vi "Untitled 1 - 22.vi"() -> ()   [LabVIEW 2016]
uses:
  Control 1.ctl
panel:
  out "I F0-ethernet 3":string
  in  "F0-ethernet 3":bool
  out "F0-e 1":bool
  out "I: PZS 2 DOP":string
  out "I: PZS 1 DOP":string
  in  "PZS 2 DOP":bool
  in  "PZS 1 DOP":bool
  out "PZS 2 DOP":bool
  out "PZS 1 DOP":bool
  out "I: BZ1K2W":string
  out "BZ1K2W":bool
  in  "BZ1K2W":bool
  out "I: DZ1K2W":string
  out "DZ1K2W":bool
  in  "DZ1K2W":bool
  out "I: F0-ethernet 4":string
  in  "F0-ethernet 4":bool
  out "F0-e 4":bool
  out "I: BZ2K2W":string
  out "I: DZ2K2W":string
  out "DZ2K2W":bool
  out "BZ2K2W":bool
  in  "BZ2K2W":bool
  in  "DZ2K2W":bool
  out "I: DZ2K1W":string
  out "DZ2K1W":bool
  in  "DZ2K1W":bool
  out "I: BZ2K1W":string
  out "BZ2K1W":bool
  in  "BZ2K1W":bool
  out "I: BZ1K1W":string
  out "BZ1K1W":bool
  in  "BZ1K1W":bool
  out "I: DZ1K1W":string
  out "DZ1K1W":bool
  in  "DZ1K1W":bool
  out "I: F0-ethernet 5":string
  in  "F0-ethernet 5":bool
  out "F0-e 5":bool
  in  "stop":T1
  out "I: BK3":string
  in  "BK3":bool
  out "BK3":bool
  in  "Delay H (0 s)":ext=100.0
  in  "BK3":bool
  in  "Delay G (0 s)":ext=100.0
  in  "BK2":bool
  out "I: BK2":string
  in  "BK 2":bool
  out "BK2":bool
  in  "Delay F (0 s)":ext=100.0
  in  "BK1":bool
  in  "BK1":bool
  out "I: BK1":string
  out "BK1":bool
  out "I F0-ethernet 2":string
  in  "Delay E (0 s)":ext=100.0
  in  "Kamera Y":bool
  out "I: Kamera Y":string
  in  "Kamera Y":bool
  out "Kamera Y":bool
  in  "F0-ethernet 2":bool
  out "F0-e 2":bool
  out "I F0-ethernet 1":string
  in  "F0-ethernet 1":bool
  out "F0-e 3":bool
  out "I: GF":string
  in  "GF":bool
  out "GF":bool
  in  "Delay D (0 s)":ext=100.0
  in  "GF":bool
  out "I: FI":string
  in  "FI":bool
  out "FI":bool
  in  "Delay C (0 s)":ext=100.0
  in  "FI":bool
  in  "F-R VISAR1":bool
  in  "Delay A (0 s)":ext=100.0
  in  "F-R VISAR 4":bool
  out "F-R VISAR 1":bool
  out "I: F-R VISAR 1":string
  in  "F-R VISAR 3":bool
  out "F-R VISAR 2":bool
  out "I: F-R VISAR 2":string
  in  "F-R VISAR2":bool
  in  "Delay B (0 s)":ext=100.0
  out "error out 2":errorcluster
  out "I 0_3":string
  in  "rele 0_6":bool
  out "read buffer 03":string
  out "0_3":bool
  out "read buffer 02":string
  out "read buffer 01":string
  out "error out":errorcluster
  out "VISA resource name out":refnum<visa-resource-name>
  in  "Trigg":bool
  in  "Setup":bool
  in  "Values start":u16(ring)=5 items=["External rising edge"=1, "Single shot internal rising edge"=3, "Single shot"=5]
  # "Current(A)"
  # "FO-ETHERNET ¹1"
  # "VISAR ¹2"
  # "VISAR ¹1"
  # "W ¹2"
  # "Current(A)"
  # "Current(A)"
  # "Current(A)"
  # "FO-ETHERNET ¹4"
  # "1 CHANAL DZ"
  # "2 CHANAL DZ"
  # "Delay (100~1099ns)"
  # "Delay (100~1099ns)"
  # "Current(A)"
  # "Current(A)"
  # "Current(A)"
  # "FO-ETHERNET ¹2"
  # "FORM IMPULSE"
  # "1 CHANAL BZ"
  # "DEEP FRONT"
  # "KAMERA Y"
  # "KAMERA B ¹1"
  # "2 CHANAL BZ"
  # "Current(A)"
  # "Current(A)"
  # "Current(A)"
  # "Current(A)"
  # "Current(A)"
  # "Current(A)"
  # "Delay (100~1099ns)"
  # "Delay (100~1099ns)"
  # "Delay (100~1099ns)"
  # "Delay (100~1099ns)"
  # "W ¹1"
  # "Current(A)"
  # "FO-ETHERNET ¹5"
  # "KAMERA B ¹2"
  # "KAMERA B ¹3"
  # "2 CHANAL DZ"
  # "1 CHANAL DZ"
  # "Current(A)"
  # "Current(A)"
  # "Current(A)"
  # "Current(A)"
  # "Current(A)"
  # "FO-ETHERNET ¹3"
  # "2 CHANAL BZ"
  # "1 CHANAL BZ"
  # "Current(A)"
  # "Current(A)"
  # "PZS ¹1"
  # "PZS ¹2"
  # "Current(A)"
  # "Current(A)"
  # "Delay (100~1099ns)"
  # "Delay (100~1099ns)"
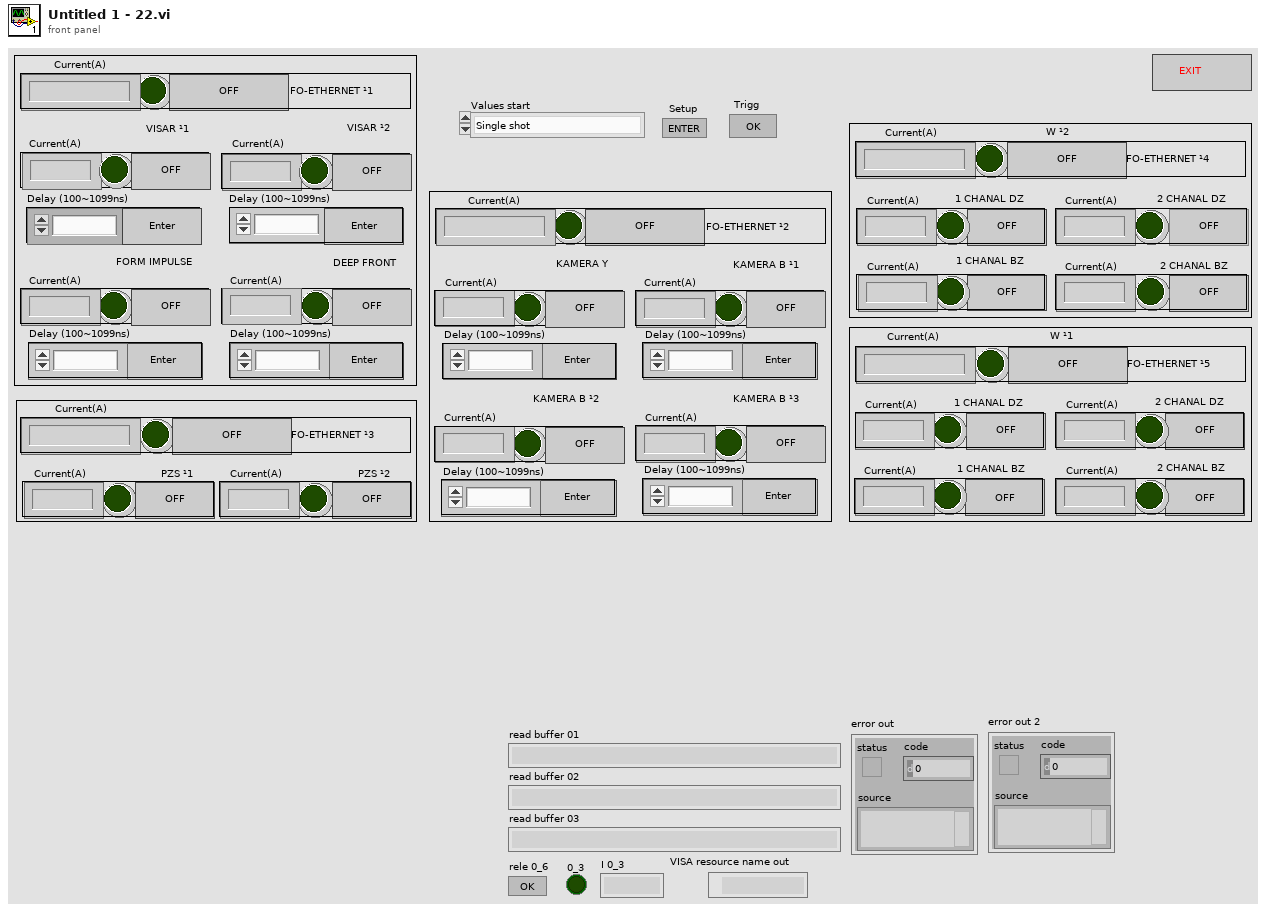
[diagram p1: front panel]
types:
  T1 = typedef "Control 1.ctl" = bool
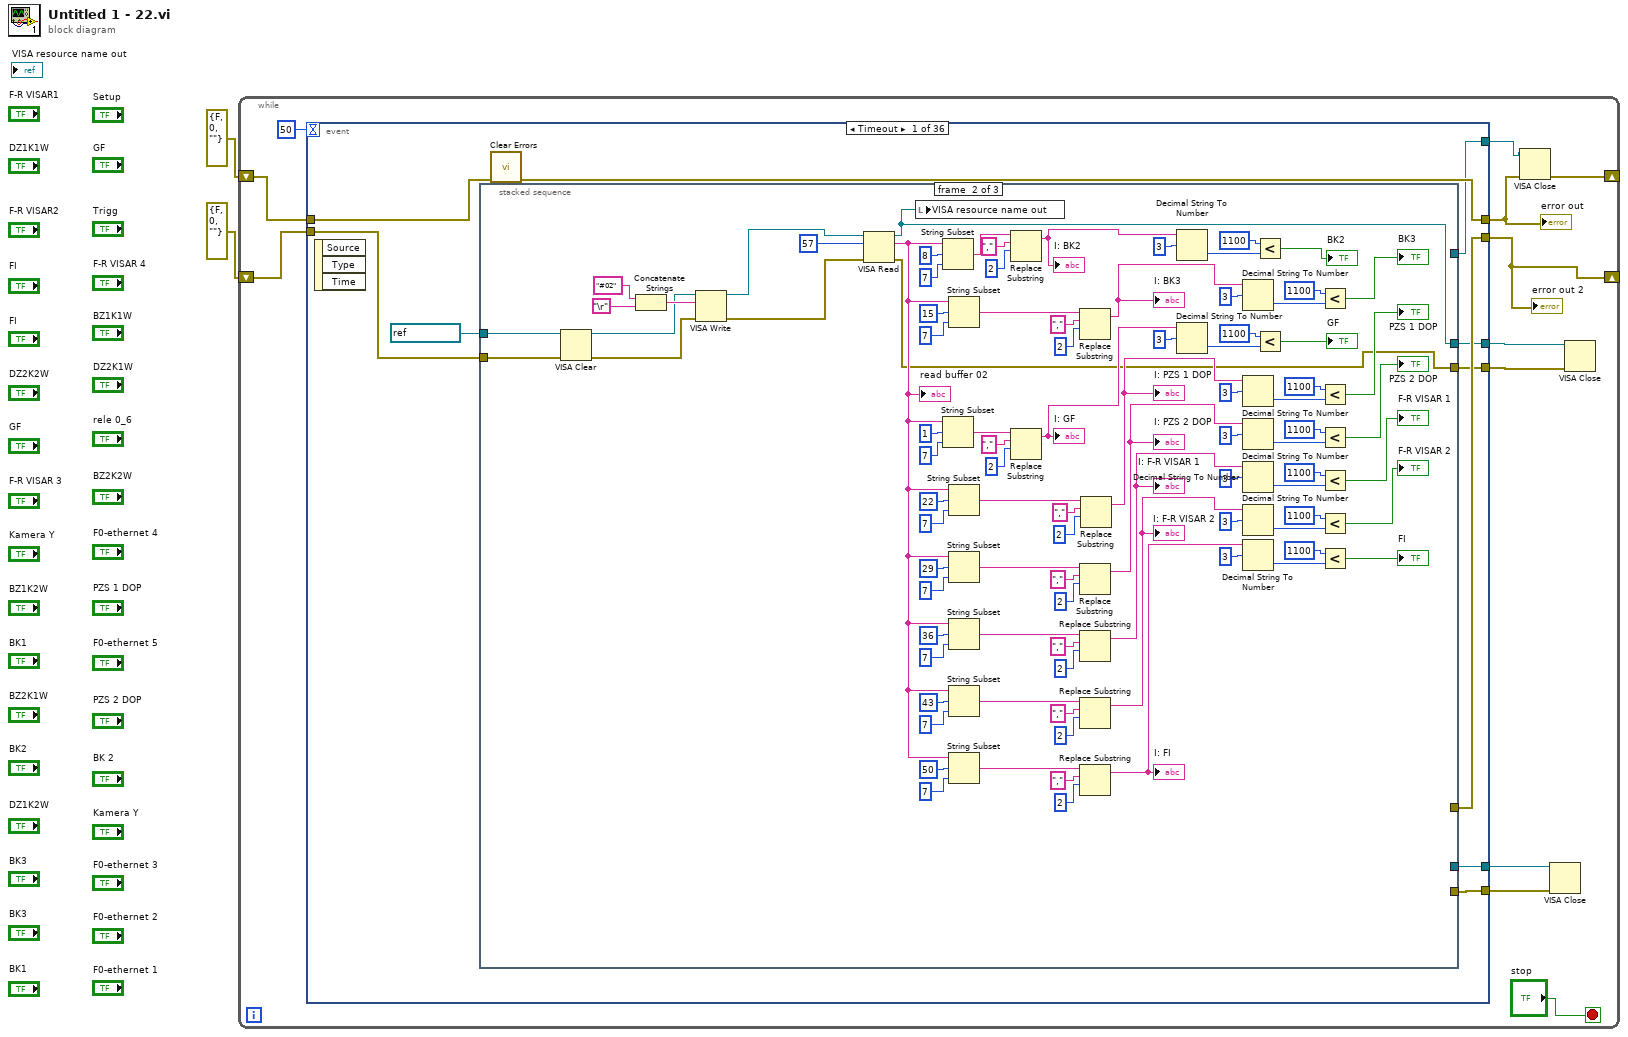
[diagram p0: block diagram]
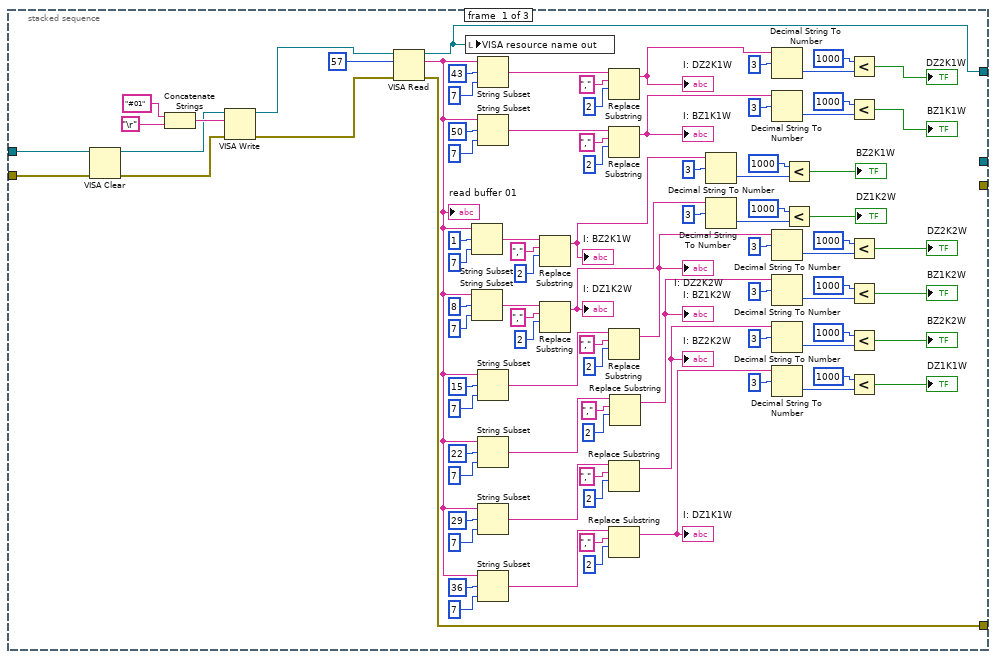
[diagram p2: hidden frame]
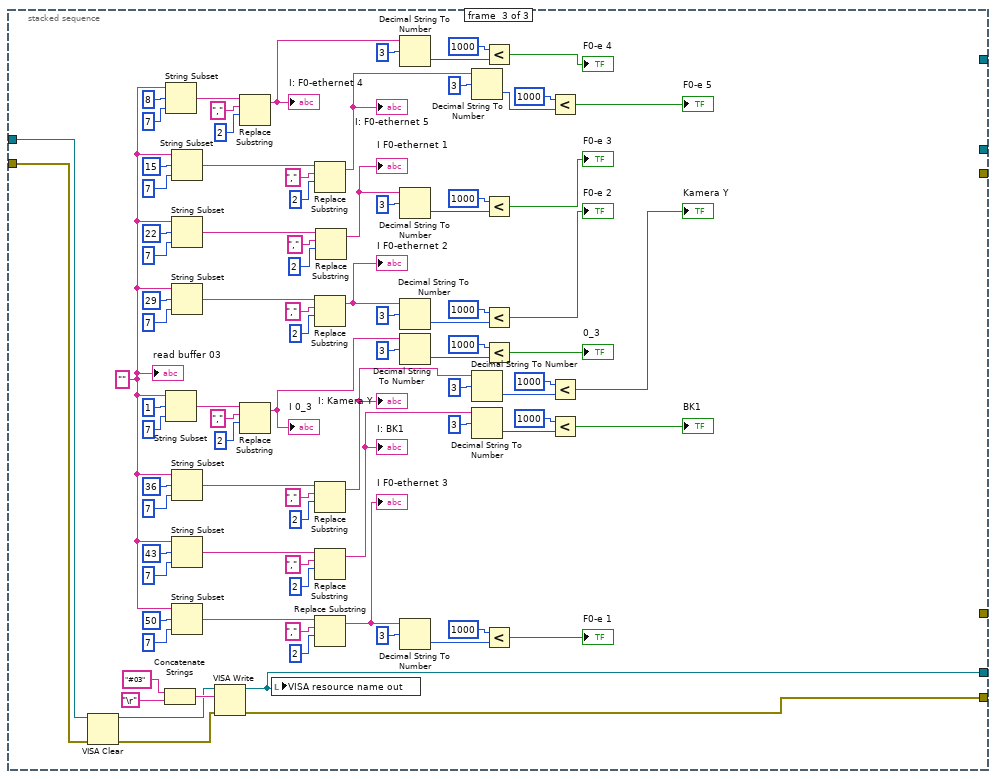
[diagram p3: hidden frame]
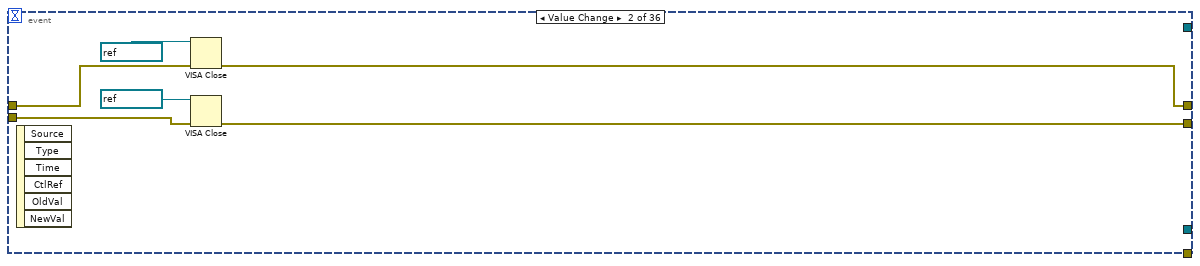
[diagram p4: hidden frame]
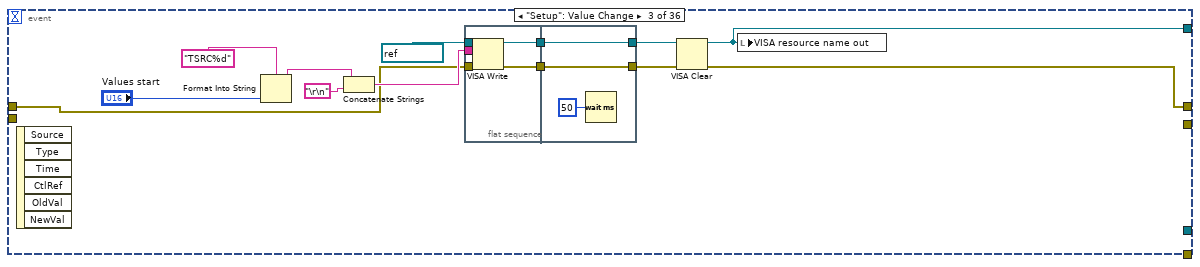
[diagram p5: hidden frame]
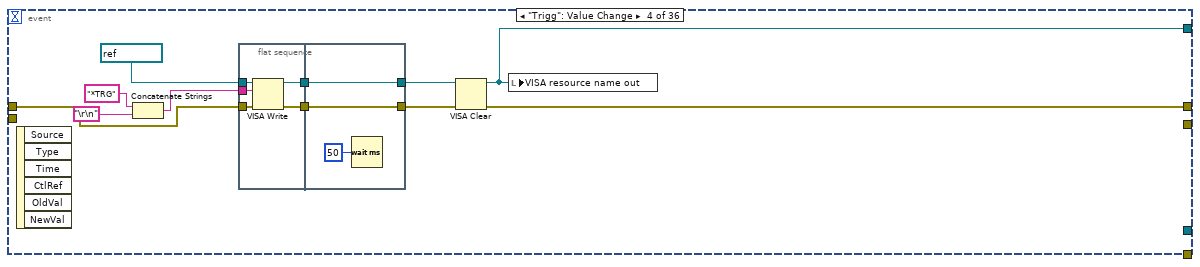
[diagram p6: hidden frame]
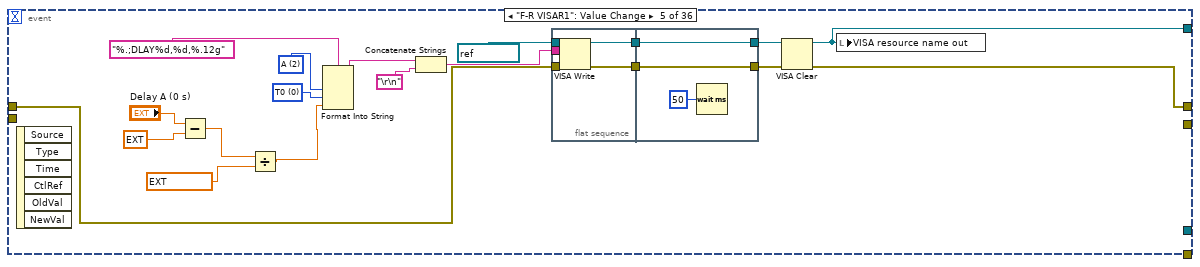
[diagram p7: hidden frame]
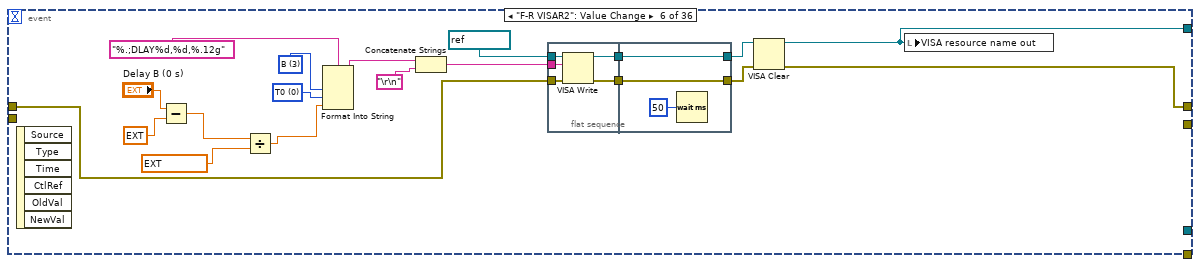
[diagram p8: hidden frame]
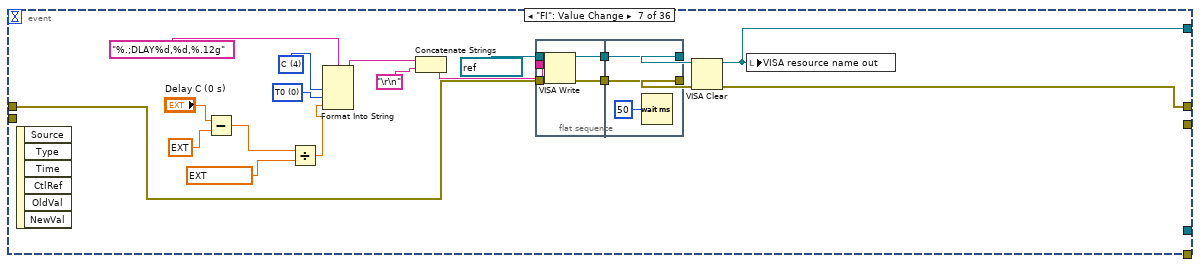
[diagram p9: hidden frame]
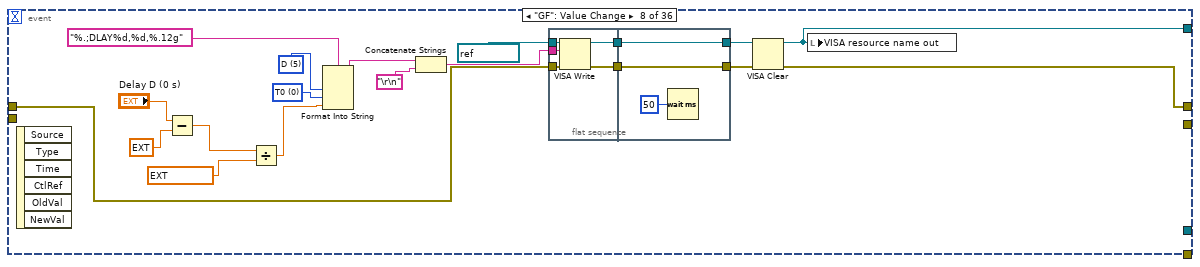
[diagram p10: hidden frame]
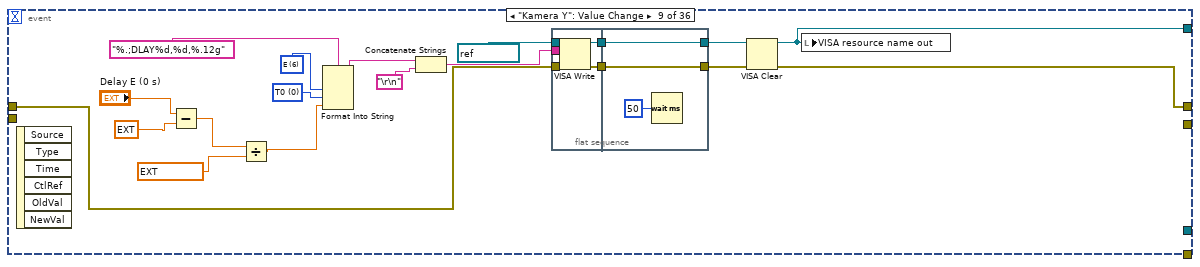
[diagram p11: hidden frame]
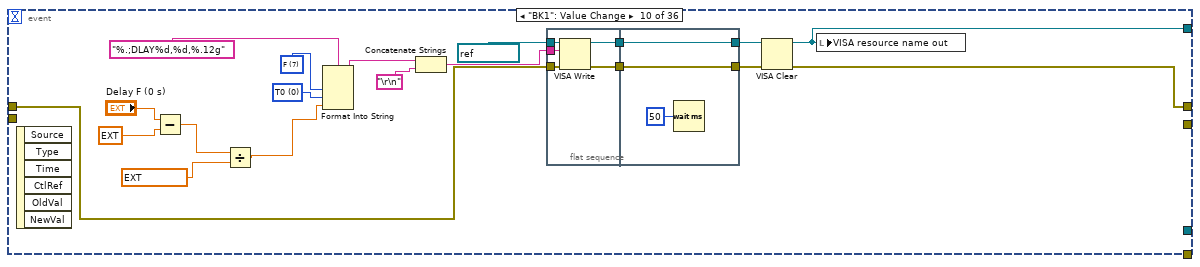
[diagram p12: hidden frame]
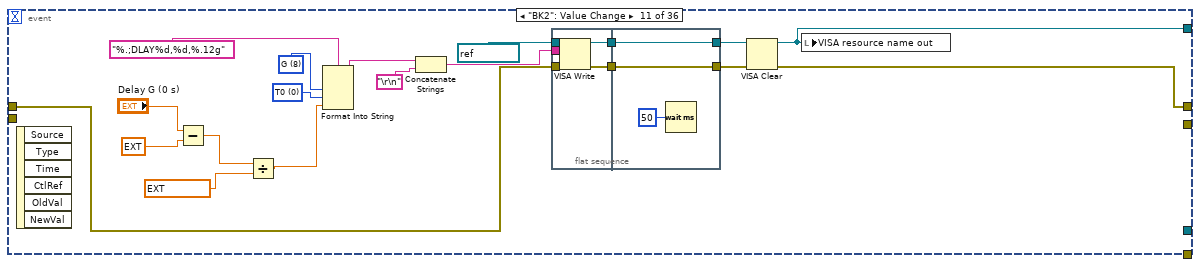
[diagram p13: hidden frame]
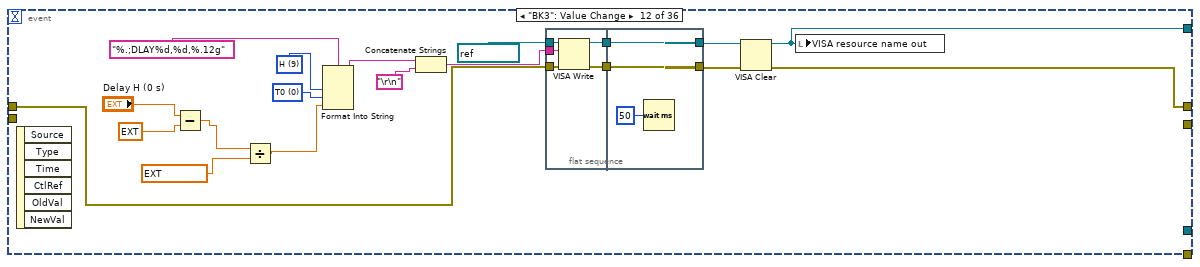
[diagram p14: hidden frame]
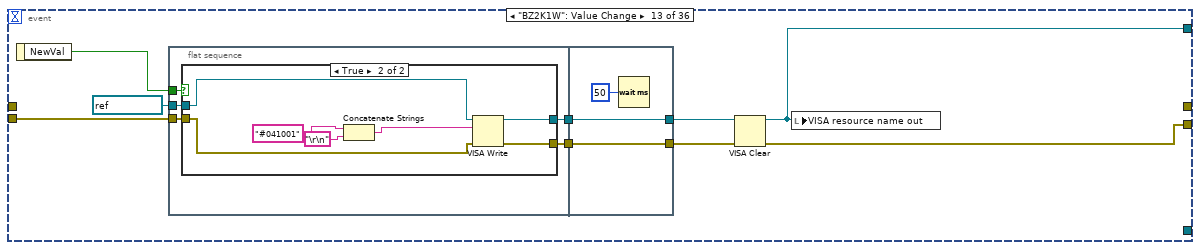
[diagram p15: hidden frame]
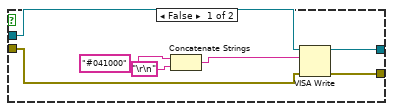
[diagram p16: hidden frame]
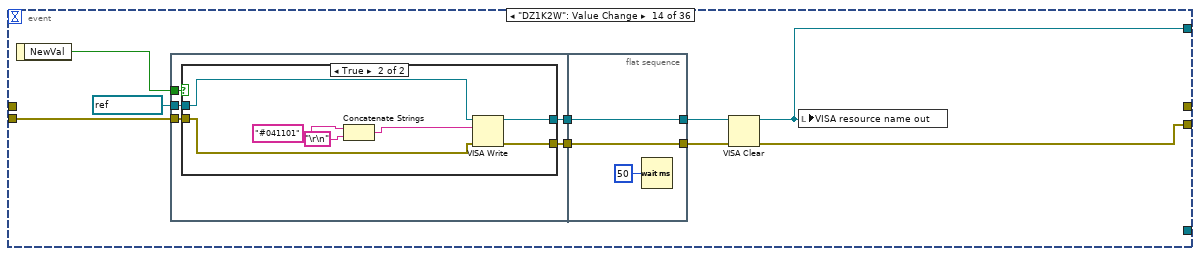
[diagram p17: hidden frame]
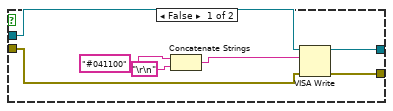
[diagram p18: hidden frame]
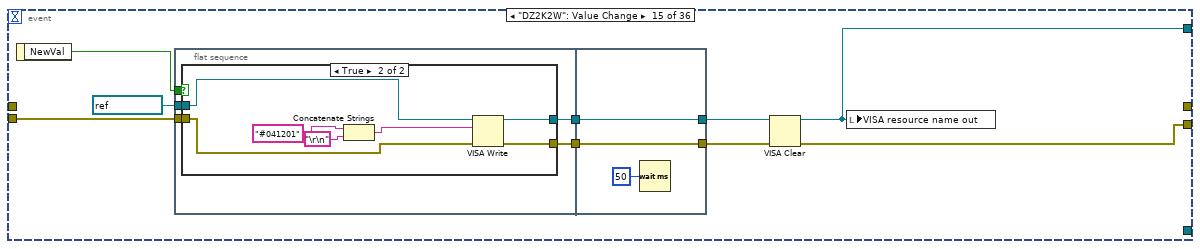
[diagram p19: hidden frame]
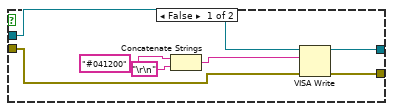
[diagram p20: hidden frame]
diagram:
  n1 = while {
    shift-right: [w11] -> _
    shift-left: errorcluster {"status"=FALSE, "code"=0, "source"=""} ("error out") -> [w14]
    shift-right: [w4] -> _
    shift-left: errorcluster {"status"=FALSE, "code"=0, "source"=""} ("error out") -> [w13]
    stop <- "stop" stop-if-true
    n2 = event shown="[0] Timeout" {
      selector: _ -> [_ _ _ _ _ _ _ _ _ _ _ _ _ _ _ _ _ _ _ _ _ _ _ _ _ _ _ _ _ _ _ _ _ _ _ _]
      dyn-events: _ -> [_ _ _ _ _ _ _ _ _ _ _ _ _ _ _ _ _ _ _ _ _ _ _ _ _ _ _ _ _ _ _ _ _ _ _ _]
      timeout: 50 -> [_ _ _ _ _ _ _ _ _ _ _ _ _ _ _ _ _ _ _ _ _ _ _ _ _ _ _ _ _ _ _ _ _ _ _ _]
      tunnel: [w23 w305 w310 w331 w356 w383 w411 w437 w464 w490 w518 w545 _ _ _ _ _ _ _ _ _ _ _ _ _ _ _ _ _ _ _ _ _ _ _ _] -> w5
      tunnel: w14 -> [w24 w306 w314 w336 w359 w386 w413 w440 w467 w494 w521 w548 _ _ _ _ _ _ _ _ _ _ _ _ _ _ _ _ _ _ _ _ _ _ _ _]
      tunnel: w13 -> [w21 w302 _ _ _ _ _ _ _ _ _ _ w570 w598 w631 w662 w693 w724 w755 w786 w817 w849 w879 w910 w941 w972 w1003 w1035 w1065 w1096 w1127 w1158 w1189 w1220 w1251 w1282]
      tunnel: [w20 w301 _ _ _ _ _ _ _ _ _ _ w566 w597 w628 w659 w691 w721 w753 w783 w814 w845 w876 w907 w938 w969 w1000 w1031 w1062 w1093 w1124 w1155 w1186 w1217 w1248 w1279] -> w4
      tunnel: [w19 _ w307 w328 w352 w379 w406 w433 w460 w487 w514 w541 w563 w594 w625 w656 w687 w718 w749 w780 w811 w842 w873 w904 w935 w966 w997 w1028 w1059 w1090 w1121 w1152 w1183 w1214 w1245 w1276] -> w10
      tunnel: [w18 _ _ _ _ _ _ _ _ _ _ _ _ _ _ _ _ _ _ _ _ _ _ _ _ _ _ _ _ _ _ _ _ _ _ _] -> w9
      tunnel: [w17 _ _ _ _ _ _ _ _ _ _ _ _ _ _ _ _ _ _ _ _ _ _ _ _ _ _ _ _ _ _ _ _ _ _ _] -> w8
      tunnel: [w16 _ _ _ _ _ _ _ _ _ _ _ _ _ _ _ _ _ _ _ _ _ _ _ _ _ _ _ _ _ _ _ _ _ _ _] -> w7
      tunnel: [w15 _ _ _ _ _ _ _ _ _ _ _ _ _ _ _ _ _ _ _ _ _ _ _ _ _ _ _ _ _ _ _ _ _ _ _] -> w6
      event Timeout {
        n3 = event-data() -> ()  [unwired: 1 in, 3 out]
        n4 = stacked-sequence {
          tunnel: refnum<visa-resource-name> "COM1" ("VISA resource name") -> [w29 w121 w234]
          tunnel: [w71 _ _] -> w20
          tunnel: w21 -> [w28 w123 w230]
          tunnel: [w25 _ _] -> w19
          tunnel: [_ w119 _] -> w18
          tunnel: [_ w118 _] -> w17
          tunnel: [_ _ w212] -> w16
          tunnel: [_ _ w211] -> w15
          frame #0 {
            n5 = VISA Clear(VISA resource name=w29, error in (no error)=w28) -> (VISA resource name out=w26:refnum<visa-resource-name>, error out=w27:errorcluster)
            n6 = Concatenate Strings("#01" ("string"), "\r") -> (w117:string)
            n7 = VISA Write(VISA resource name=w26, write buffer=w117, error in (no error)=w27) -> (VISA resource name out=w74:refnum<visa-resource-name>, error out=w73:errorcluster)  [unwired: 1 out]
            n8 = VISA Read(VISA resource name=w74, byte count=u32 57, error in (no error)=w73) -> (VISA resource name out=w25:refnum<visa-resource-name>, read buffer=w46:string, error out=w71:errorcluster)  [unwired: 1 out]
            "read buffer 01" <- w46
            n9 = local write "VISA resource name out"(w25) -> ()
            n10 = String Subset(string=w46, offset (0)=1, length (rest)=7 ("length (rest)")) -> (substring=w91:string)
            n11 = String Subset(string=w46, offset (0)=8, length (rest)=7 ("length (rest)")) -> (substring=w96:string)
            n12 = String Subset(string=w46, offset (0)=43, length (rest)=7 ("length (rest)")) -> (substring=w111:string)
            n13 = String Subset(string=w46, offset (0)=50, length (rest)=7 ("length (rest)")) -> (substring=w114:string)
            n14 = String Subset(string=w46, offset (0)=15, length (rest)=7 ("length (rest)")) -> (substring=w99:string)
            n15 = String Subset(string=w46, offset (0)=22, length (rest)=7 ("length (rest)")) -> (substring=w102:string)
            n16 = String Subset(string=w46, offset (0)=29, length (rest)=7 ("length (rest)")) -> (substring=w105:string)
            n17 = String Subset(string=w46, offset (0)=36, length (rest)=7 ("length (rest)")) -> (substring=w108:string)
            n18 = Replace Substring(3:2 ("offset (0)"), 4:"," ("substring (\"\")"), 5:w91) -> (1:w45:string)  [unwired: 1 in, 1 out]
            "I: BZ2K1W" <- w45
            n19 = Replace Substring(3:2 ("offset (0)"), 4:"," ("substring (\"\")"), 5:w96) -> (1:w43:string)  [unwired: 1 in, 1 out]
            "I: DZ1K2W" <- w43
            n20 = Replace Substring(3:2 ("offset (0)"), 4:"," ("substring (\"\")"), 5:w111) -> (1:w32:string)  [unwired: 1 in, 1 out]
            "I: DZ2K1W" <- w32
            n21 = Replace Substring(3:2 ("offset (0)"), 4:"," ("substring (\"\")"), 5:w114) -> (1:w31:string)  [unwired: 1 in, 1 out]
            "I: BZ1K1W" <- w31
            n22 = Replace Substring(3:2 ("offset (0)"), 4:"," ("substring (\"\")"), 5:w99) -> (1:w41:string)  [unwired: 1 in, 1 out]
            "I: DZ2K2W" <- w41
            n23 = Replace Substring(3:2 ("offset (0)"), 4:"," ("substring (\"\")"), 5:w105) -> (1:w37:string)  [unwired: 1 in, 1 out]
            "I: BZ2K2W" <- w37
            n24 = Replace Substring(3:2 ("offset (0)"), 4:"," ("substring (\"\")"), 5:w108) -> (1:w34:string)  [unwired: 1 in, 1 out]
            "I: DZ1K1W" <- w34
            n25 = Replace Substring(3:2 ("offset (0)"), 4:"," ("substring (\"\")"), 5:w102) -> (1:w39:string)  [unwired: 1 in, 1 out]
            "I: BZ1K2W" <- w39
            n26 = Decimal String To Number(string=w45, offset=3) -> (number=w54:i32)  [unwired: 1 in, 1 out]
            n27 = Decimal String To Number(string=w43, offset=3) -> (number=w57:i32)  [unwired: 1 in, 1 out]
            n28 = Decimal String To Number(string=w32, offset=3) -> (number=w51:i32)  [unwired: 1 in, 1 out]
            n29 = Decimal String To Number(string=w31, offset=3) -> (number=w48:i32)  [unwired: 1 in, 1 out]
            n30 = Decimal String To Number(string=w41, offset=3) -> (number=w60:i32)  [unwired: 1 in, 1 out]
            n31 = Decimal String To Number(string=w39, offset=3) -> (number=w63:i32)  [unwired: 1 in, 1 out]
            n32 = Decimal String To Number(string=w37, offset=3) -> (number=w66:i32)  [unwired: 1 in, 1 out]
            n33 = Decimal String To Number(string=w34, offset=3) -> (number=w69:i32)  [unwired: 1 in, 1 out]
            n34 = Less?(x=1000, y=w54) -> (x < y?=→"BZ2K1W":bool)
            n35 = Less?(x=1000, y=w57) -> (x < y?=→"DZ1K2W":bool)
            n36 = Less?(x=1000, y=w51) -> (x < y?=→"DZ2K1W":bool)
            n37 = Less?(x=1000, y=w48) -> (x < y?=→"BZ1K1W":bool)
            n38 = Less?(x=1000, y=w60) -> (x < y?=→"DZ2K2W":bool)
            n39 = Less?(x=1000, y=w63) -> (x < y?=→"BZ1K2W":bool)
            n40 = Less?(x=1000, y=w66) -> (x < y?=→"BZ2K2W":bool)
            n41 = Less?(x=1000, y=w69) -> (x < y?=→"DZ1K1W":bool)
          }
          frame #1 {
            n42 = VISA Clear(VISA resource name=w121, error in (no error)=w123) -> (VISA resource name out=w120:refnum<visa-resource-name>, error out=w122:errorcluster)
            n43 = Concatenate Strings("#02" ("string"), "\r") -> (w210:string)
            n44 = VISA Write(VISA resource name=w120, write buffer=w210, error in (no error)=w122) -> (VISA resource name out=w167:refnum<visa-resource-name>, error out=w166:errorcluster)  [unwired: 1 out]
            n45 = VISA Read(VISA resource name=w167, byte count=u32 57, error in (no error)=w166) -> (VISA resource name out=w119:refnum<visa-resource-name>, read buffer=w140:string, error out=w118:errorcluster)  [unwired: 1 out]
            "read buffer 02" <- w140
            n46 = local write "VISA resource name out"(w119) -> ()
            n47 = String Subset(string=w140, offset (0)=8, length (rest)=7 ("length (rest)")) -> (substring=w189:string)
            n48 = String Subset(string=w140, offset (0)=1, length (rest)=7 ("length (rest)")) -> (substring=w184:string)
            n49 = String Subset(string=w140, offset (0)=15, length (rest)=7 ("length (rest)")) -> (substring=w192:string)
            n50 = String Subset(string=w140, offset (0)=22, length (rest)=7 ("length (rest)")) -> (substring=w195:string)
            n51 = String Subset(string=w140, offset (0)=29, length (rest)=7 ("length (rest)")) -> (substring=w198:string)
            n52 = String Subset(string=w140, offset (0)=36, length (rest)=7 ("length (rest)")) -> (substring=w201:string)
            n53 = String Subset(string=w140, offset (0)=43, length (rest)=7 ("length (rest)")) -> (substring=w204:string)
            n54 = String Subset(string=w140, offset (0)=50, length (rest)=7 ("length (rest)")) -> (substring=w207:string)
            n55 = Replace Substring(3:2 ("offset (0)"), 4:"," ("substring (\"\")"), 5:w189) -> (1:w136:string)  [unwired: 1 in, 1 out]
            "I: BK2" <- w136
            n56 = Replace Substring(3:2 ("offset (0)"), 4:"," ("substring (\"\")"), 5:w184) -> (1:w138:string)  [unwired: 1 in, 1 out]
            "I: GF" <- w138
            n57 = Replace Substring(3:2 ("offset (0)"), 4:"," ("substring (\"\")"), 5:w192) -> (1:w135:string)  [unwired: 1 in, 1 out]
            "I: BK3" <- w135
            n58 = Replace Substring(3:2 ("offset (0)"), 4:"," ("substring (\"\")"), 5:w198) -> (1:w130:string)  [unwired: 1 in, 1 out]
            "I: PZS 2 DOP" <- w130
            n59 = Replace Substring(3:2 ("offset (0)"), 4:"," ("substring (\"\")"), 5:w201) -> (1:w128:string)  [unwired: 1 in, 1 out]
            "I: F-R VISAR 1" <- w128
            n60 = Replace Substring(3:2 ("offset (0)"), 4:"," ("substring (\"\")"), 5:w204) -> (1:w127:string)  [unwired: 1 in, 1 out]
            "I: F-R VISAR 2" <- w127
            n61 = Replace Substring(3:2 ("offset (0)"), 4:"," ("substring (\"\")"), 5:w207) -> (1:w126:string)  [unwired: 1 in, 1 out]
            "I: FI" <- w126
            n62 = Replace Substring(3:2 ("offset (0)"), 4:"," ("substring (\"\")"), 5:w195) -> (1:w133:string)  [unwired: 1 in, 1 out]
            "I: PZS 1 DOP" <- w133
            n63 = Decimal String To Number(string=w136, offset=3) -> (number=w151:i32)  [unwired: 1 in, 1 out]
            n64 = Decimal String To Number(string=w138, offset=3) -> (number=w148:i32)  [unwired: 1 in, 1 out]
            n65 = Decimal String To Number(string=w135, offset=3) -> (number=w154:i32)  [unwired: 1 in, 1 out]
            n66 = Decimal String To Number(string=w133, offset=3) -> (number=w157:i32)  [unwired: 1 in, 1 out]
            n67 = Decimal String To Number(string=w130, offset=3) -> (number=w160:i32)  [unwired: 1 in, 1 out]
            n68 = Decimal String To Number(string=w128, offset=3) -> (number=w163:i32)  [unwired: 1 in, 1 out]
            n69 = Decimal String To Number(string=w127, offset=3) -> (number=w145:i32)  [unwired: 1 in, 1 out]
            n70 = Decimal String To Number(string=w126, offset=3) -> (number=w142:i32)  [unwired: 1 in, 1 out]
            n71 = Less?(x=1100, y=w151) -> (x < y?=→"BK2":bool)
            n72 = Less?(x=1100, y=w148) -> (x < y?=→"GF":bool)
            n73 = Less?(x=1100, y=w154) -> (x < y?=→"BK3":bool)
            n74 = Less?(x=1100, y=w157) -> (x < y?=→"PZS 1 DOP":bool)
            n75 = Less?(x=1100, y=w160) -> (x < y?=→"PZS 2 DOP":bool)
            n76 = Less?(x=1100, y=w163) -> (x < y?=→"F-R VISAR 1":bool)
            n77 = Less?(x=1100, y=w145) -> (x < y?=→"F-R VISAR 2":bool)
            n78 = Less?(x=1100, y=w142) -> (x < y?=→"FI":bool)
          }
          frame #2 {
            w229 = "" ("string")
            n79 = VISA Clear(VISA resource name=w234, error in (no error)=w230) -> (VISA resource name out=w232:refnum<visa-resource-name>, error out=w233:errorcluster)
            n80 = Concatenate Strings("#03" ("string"), "\r") -> (w300:string)
            n81 = String Subset(string=w229, offset (0)=8, length (rest)=7 ("length (rest)")) -> (substring=w279:string)
            n82 = String Subset(string=w229, offset (0)=1, length (rest)=7 ("length (rest)")) -> (substring=w231:string)
            n83 = String Subset(string=w229, offset (0)=15, length (rest)=7 ("length (rest)")) -> (substring=w282:string)
            n84 = String Subset(string=w229, offset (0)=22, length (rest)=7 ("length (rest)")) -> (substring=w285:string)
            n85 = String Subset(string=w229, offset (0)=29, length (rest)=7 ("length (rest)")) -> (substring=w288:string)
            n86 = String Subset(string=w229, offset (0)=36, length (rest)=7 ("length (rest)")) -> (substring=w291:string)
            n87 = String Subset(string=w229, offset (0)=43, length (rest)=7 ("length (rest)")) -> (substring=w294:string)
            n88 = String Subset(string=w229, offset (0)=50, length (rest)=7 ("length (rest)")) -> (substring=w297:string)
            n89 = VISA Write(VISA resource name=w232, write buffer=w300, error in (no error)=w233) -> (VISA resource name out=w211:refnum<visa-resource-name>, error out=w212:errorcluster)  [unwired: 1 out]
            n90 = Replace Substring(3:2 ("offset (0)"), 4:"," ("substring (\"\")"), 5:w279) -> (1:w226:string)  [unwired: 1 in, 1 out]
            "I: F0-ethernet 4" <- w226
            n91 = Replace Substring(3:2 ("offset (0)"), 4:"," ("substring (\"\")"), 5:w231) -> (1:w228:string)  [unwired: 1 in, 1 out]
            "I 0_3" <- w228
            n92 = local write "VISA resource name out"(w211) -> ()
            n93 = Replace Substring(3:2 ("offset (0)"), 4:"," ("substring (\"\")"), 5:w282) -> (1:w224:string)  [unwired: 1 in, 1 out]
            "I: F0-ethernet 5" <- w224
            n94 = Replace Substring(3:2 ("offset (0)"), 4:"," ("substring (\"\")"), 5:w288) -> (1:w219:string)  [unwired: 1 in, 1 out]
            "I F0-ethernet 2" <- w219
            n95 = Replace Substring(3:2 ("offset (0)"), 4:"," ("substring (\"\")"), 5:w291) -> (1:w217:string)  [unwired: 1 in, 1 out]
            "I: Kamera Y" <- w217
            n96 = Replace Substring(3:2 ("offset (0)"), 4:"," ("substring (\"\")"), 5:w294) -> (1:w215:string)  [unwired: 1 in, 1 out]
            "I: BK1" <- w215
            n97 = Replace Substring(3:2 ("offset (0)"), 4:"," ("substring (\"\")"), 5:w297) -> (1:w213:string)  [unwired: 1 in, 1 out]
            "I F0-ethernet 3" <- w213
            n98 = Replace Substring(3:2 ("offset (0)"), 4:"," ("substring (\"\")"), 5:w285) -> (1:w222:string)  [unwired: 1 in, 1 out]
            "I F0-ethernet 1" <- w222
            n99 = Decimal String To Number(string=w226, offset=3) -> (number=w245:i32)  [unwired: 1 in, 1 out]
            n100 = Decimal String To Number(string=w222, offset=3) -> (number=w251:i32)  [unwired: 1 in, 1 out]
            n101 = Decimal String To Number(string=w219, offset=3) -> (number=w254:i32)  [unwired: 1 in, 1 out]
            n102 = Decimal String To Number(string=w228, offset=3) -> (number=w242:i32)  [unwired: 1 in, 1 out]
            n103 = Decimal String To Number(string=w213, offset=3) -> (number=w236:i32)  [unwired: 1 in, 1 out]
            n104 = Decimal String To Number(string=w224, offset=3) -> (number=w248:i32)  [unwired: 1 in, 1 out]
            n105 = Decimal String To Number(string=w217, offset=3) -> (number=w257:i32)  [unwired: 1 in, 1 out]
            n106 = Decimal String To Number(string=w215, offset=3) -> (number=w239:i32)  [unwired: 1 in, 1 out]
            n107 = Less?(x=1000, y=w245) -> (x < y?=→"F0-e 4":bool)
            n108 = Less?(x=1000, y=w251) -> (x < y?=→"F0-e 3":bool)
            n109 = Less?(x=1000, y=w254) -> (x < y?=→"F0-e 2":bool)
            n110 = Less?(x=1000, y=w242) -> (x < y?=→"0_3":bool)
            n111 = Less?(x=1000, y=w236) -> (x < y?=→"F0-e 1":bool)
            n112 = Less?(x=1000, y=w248) -> (x < y?=→"F0-e 5":bool)
            n113 = Less?(x=1000, y=w257) -> (x < y?=→"Kamera Y":bool)
            n114 = Less?(x=1000, y=w239) -> (x < y?=→"BK1":bool)
            "read buffer 03" <- w229
          }
        }
        n115 = call <vilib>:"Clear Errors.vi"("error in (no error)"=w24) -> ("error out"=w23:errorcluster)  [unwired: 5 in, 1 out]
      }
      event Value Change {
        n116 = event-data() -> ()  [unwired: 1 in, 6 out]
        n117 = VISA Close(VISA resource name=refnum<visa-resource-name> "DG645", error in (no error)=w306) -> (error out=w305:errorcluster)
        n118 = VISA Close(VISA resource name=refnum<visa-resource-name> "COM1", error in (no error)=w302) -> (error out=w301:errorcluster)
      }
      event "Setup": Value Change {
        n119 = event-data() -> ()  [unwired: 1 in, 6 out]
        n120 = Format Into String(format string="TSRC%d", "Values start") -> (resulting string=w317:string)  [unwired: 2 in, 1 out]
        n121 = Concatenate Strings(w317, "\r\n") -> (w319:string)
        n122 = flat-sequence {
          tunnel: w319 -> [w324]
          tunnel: w314 -> [w323]
          tunnel: refnum<visa-resource-name> "DG645" ("VISA resource name") -> [w322]
          tunnel: [w321] -> w309
          tunnel: [w320] -> w308
          tunnel: [w326] -> w311
          tunnel: [w327] -> w312
          tunnel: w309 -> [w327]
          tunnel: w308 -> [w326]
          frame #0 {
            n123 = VISA Write(VISA resource name=w322, write buffer=w324, error in (no error)=w323) -> (VISA resource name out=w320:refnum<visa-resource-name>, error out=w321:errorcluster)  [unwired: 1 out]
          }
          frame #1 {
            n124 = Wait (ms)(milliseconds to wait=u32 50) -> ()  [unwired: 1 out]
          }
        }
        n125 = VISA Clear(VISA resource name=w311, error in (no error)=w312) -> (VISA resource name out=w307:refnum<visa-resource-name>, error out=w310:errorcluster)
        n126 = local write "VISA resource name out"(w307) -> ()
      }
      event "Trigg": Value Change {
        n127 = event-data() -> ()  [unwired: 1 in, 6 out]
        n128 = Concatenate Strings("*TRG" ("string"), "\r\n") -> (w337:string)
        n129 = flat-sequence {
          tunnel: w337 -> [w343]
          tunnel: w336 -> [w342]
          tunnel: refnum<visa-resource-name> "DG645" ("VISA resource name") -> [w341]
          tunnel: [w340] -> w330
          tunnel: [w339] -> w329
          tunnel: [w345] -> w332
          tunnel: [w346] -> w333
          tunnel: w330 -> [w346]
          tunnel: w329 -> [w345]
          frame #0 {
            n130 = VISA Write(VISA resource name=w341, write buffer=w343, error in (no error)=w342) -> (VISA resource name out=w339:refnum<visa-resource-name>, error out=w340:errorcluster)  [unwired: 1 out]
          }
          frame #1 {
            n131 = Wait (ms)(milliseconds to wait=u32 50) -> ()  [unwired: 1 out]
          }
        }
        n132 = VISA Clear(VISA resource name=w332, error in (no error)=w333) -> (VISA resource name out=w328:refnum<visa-resource-name>, error out=w331:errorcluster)
        n133 = local write "VISA resource name out"(w328) -> ()
      }
      event "F-R VISAR1": Value Change {
        w360 = u16 0 items=["T0"=0, "A"=2, "B"=3, "C"=4, "D"=5, "E"=6, "F"=7, "G"=8, "H"=9] ("Reference Channel (0:T0)")
        w364 = u16 2 items=["A"=2, "B"=3, "C"=4, "D"=5, "E"=6, "F"=7, "G"=8, "H"=9] ("Channel to Modify (2:A)")
        n134 = event-data() -> ()  [unwired: 1 in, 6 out]
        n135 = Subtract(x="Delay A (0 s)", y=ext 100.0) -> (x-y=w347:ext)
        n136 = Divide(x=w347, y=ext 1000000000.0) -> (x/y=w350:ext)
        n137 = Format Into String(format string="%.;DLAY%d,%d,%.12g" ("Set Delay Command"), w364, w360, w350) -> (resulting string=w363:string)  [unwired: 2 in, 1 out]
        n138 = Concatenate Strings(w363, "\r\n") -> (w362:string)
        n139 = flat-sequence {
          tunnel: w362 -> [w370]
          tunnel: w359 -> [w369]
          tunnel: refnum<visa-resource-name> "DG645" ("VISA resource name") -> [w368]
          tunnel: [w367] -> w354
          tunnel: [w366] -> w353
          tunnel: [w372] -> w355
          tunnel: [w373] -> w357
          tunnel: w354 -> [w373]
          tunnel: w353 -> [w372]
          frame #0 {
            n140 = VISA Write(VISA resource name=w368, write buffer=w370, error in (no error)=w369) -> (VISA resource name out=w366:refnum<visa-resource-name>, error out=w367:errorcluster)  [unwired: 1 out]
          }
          frame #1 {
            n141 = Wait (ms)(milliseconds to wait=u32 50) -> ()  [unwired: 1 out]
          }
        }
        n142 = VISA Clear(VISA resource name=w355, error in (no error)=w357) -> (VISA resource name out=w352:refnum<visa-resource-name>, error out=w356:errorcluster)
        n143 = local write "VISA resource name out"(w352) -> ()
      }
      event "F-R VISAR2": Value Change {
        w387 = u16 0 items=["T0"=0, "A"=2, "B"=3, "C"=4, "D"=5, "E"=6, "F"=7, "G"=8, "H"=9] ("Reference Channel (0:T0)")
        w391 = u16 3 items=["A"=2, "B"=3, "C"=4, "D"=5, "E"=6, "F"=7, "G"=8, "H"=9] ("Channel to Modify (2:A)")
        n144 = event-data() -> ()  [unwired: 1 in, 6 out]
        n145 = Subtract(x="Delay B (0 s)", y=ext 100.0) -> (x-y=w374:ext)
        n146 = Divide(x=w374, y=ext 1000000000.0) -> (x/y=w377:ext)
        n147 = Format Into String(format string="%.;DLAY%d,%d,%.12g" ("Set Delay Command"), w391, w387, w377) -> (resulting string=w390:string)  [unwired: 2 in, 1 out]
        n148 = Concatenate Strings(w390, "\r\n") -> (w389:string)
        n149 = flat-sequence {
          tunnel: w389 -> [w397]
          tunnel: w386 -> [w396]
          tunnel: refnum<visa-resource-name> "DG645" ("VISA resource name") -> [w395]
          tunnel: [w394] -> w381
          tunnel: [w393] -> w380
          tunnel: [w399] -> w382
          tunnel: [w400] -> w384
          tunnel: w381 -> [w400]
          tunnel: w380 -> [w399]
          frame #0 {
            n150 = VISA Write(VISA resource name=w395, write buffer=w397, error in (no error)=w396) -> (VISA resource name out=w393:refnum<visa-resource-name>, error out=w394:errorcluster)  [unwired: 1 out]
          }
          frame #1 {
            n151 = Wait (ms)(milliseconds to wait=u32 50) -> ()  [unwired: 1 out]
          }
        }
        n152 = VISA Clear(VISA resource name=w382, error in (no error)=w384) -> (VISA resource name out=w379:refnum<visa-resource-name>, error out=w383:errorcluster)
        n153 = local write "VISA resource name out"(w379) -> ()
      }
      event "FI": Value Change {
        w414 = u16 0 items=["T0"=0, "A"=2, "B"=3, "C"=4, "D"=5, "E"=6, "F"=7, "G"=8, "H"=9] ("Reference Channel (0:T0)")
        w418 = u16 4 items=["A"=2, "B"=3, "C"=4, "D"=5, "E"=6, "F"=7, "G"=8, "H"=9] ("Channel to Modify (2:A)")
        n154 = event-data() -> ()  [unwired: 1 in, 6 out]
        n155 = Subtract(x="Delay C (0 s)", y=ext 100.0) -> (x-y=w402:ext)
        n156 = Divide(x=w402, y=ext 1000000000.0) -> (x/y=w403:ext)
        n157 = Format Into String(format string="%.;DLAY%d,%d,%.12g" ("Set Delay Command"), w418, w414, w403) -> (resulting string=w417:string)  [unwired: 2 in, 1 out]
        n158 = Concatenate Strings(w417, "\r\n") -> (w416:string)
        n159 = flat-sequence {
          tunnel: w416 -> [w424]
          tunnel: w413 -> [w423]
          tunnel: refnum<visa-resource-name> "DG645" ("VISA resource name") -> [w422]
          tunnel: [w421] -> w408
          tunnel: [w420] -> w407
          tunnel: [w426] -> w409
          tunnel: [w427] -> w410
          tunnel: w408 -> [w427]
          tunnel: w407 -> [w426]
          frame #0 {
            n160 = VISA Write(VISA resource name=w422, write buffer=w424, error in (no error)=w423) -> (VISA resource name out=w420:refnum<visa-resource-name>, error out=w421:errorcluster)  [unwired: 1 out]
          }
          frame #1 {
            n161 = Wait (ms)(milliseconds to wait=u32 50) -> ()  [unwired: 1 out]
          }
        }
        n162 = VISA Clear(VISA resource name=w409, error in (no error)=w410) -> (VISA resource name out=w406:refnum<visa-resource-name>, error out=w411:errorcluster)
        n163 = local write "VISA resource name out"(w406) -> ()
      }
      event "GF": Value Change {
        w441 = u16 0 items=["T0"=0, "A"=2, "B"=3, "C"=4, "D"=5, "E"=6, "F"=7, "G"=8, "H"=9] ("Reference Channel (0:T0)")
        w445 = u16 5 items=["A"=2, "B"=3, "C"=4, "D"=5, "E"=6, "F"=7, "G"=8, "H"=9] ("Channel to Modify (2:A)")
        n164 = event-data() -> ()  [unwired: 1 in, 6 out]
        n165 = Subtract(x="Delay D (0 s)", y=ext 100.0) -> (x-y=w430:ext)
        n166 = Divide(x=w430, y=ext 1000000000.0) -> (x/y=w428:ext)
        n167 = Format Into String(format string="%.;DLAY%d,%d,%.12g" ("Set Delay Command"), w445, w441, w428) -> (resulting string=w444:string)  [unwired: 2 in, 1 out]
        n168 = Concatenate Strings(w444, "\r\n") -> (w443:string)
        n169 = flat-sequence {
          tunnel: w443 -> [w451]
          tunnel: w440 -> [w450]
          tunnel: refnum<visa-resource-name> "DG645" ("VISA resource name") -> [w449]
          tunnel: [w448] -> w435
          tunnel: [w447] -> w434
          tunnel: [w453] -> w436
          tunnel: [w454] -> w438
          tunnel: w435 -> [w454]
          tunnel: w434 -> [w453]
          frame #0 {
            n170 = VISA Write(VISA resource name=w449, write buffer=w451, error in (no error)=w450) -> (VISA resource name out=w447:refnum<visa-resource-name>, error out=w448:errorcluster)  [unwired: 1 out]
          }
          frame #1 {
            n171 = Wait (ms)(milliseconds to wait=u32 50) -> ()  [unwired: 1 out]
          }
        }
        n172 = VISA Clear(VISA resource name=w436, error in (no error)=w438) -> (VISA resource name out=w433:refnum<visa-resource-name>, error out=w437:errorcluster)
        n173 = local write "VISA resource name out"(w433) -> ()
      }
      event "Kamera Y": Value Change {
        w468 = u16 0 items=["T0"=0, "A"=2, "B"=3, "C"=4, "D"=5, "E"=6, "F"=7, "G"=8, "H"=9] ("Reference Channel (0:T0)")
        w472 = u16 6 items=["A"=2, "B"=3, "C"=4, "D"=5, "E"=6, "F"=7, "G"=8, "H"=9] ("Channel to Modify (2:A)")
        n174 = event-data() -> ()  [unwired: 1 in, 6 out]
        n175 = Subtract(x="Delay E (0 s)", y=ext 100.0) -> (x-y=w456:ext)
        n176 = Divide(x=w456, y=ext 1000000000.0) -> (x/y=w455:ext)
        n177 = Format Into String(format string="%.;DLAY%d,%d,%.12g" ("Set Delay Command"), w472, w468, w455) -> (resulting string=w471:string)  [unwired: 2 in, 1 out]
        n178 = Concatenate Strings(w471, "\r\n") -> (w470:string)
        n179 = flat-sequence {
          tunnel: w470 -> [w478]
          tunnel: w467 -> [w477]
          tunnel: refnum<visa-resource-name> "DG645" ("VISA resource name") -> [w476]
          tunnel: [w475] -> w462
          tunnel: [w474] -> w461
          tunnel: [w480] -> w463
          tunnel: [w481] -> w465
          tunnel: w462 -> [w481]
          tunnel: w461 -> [w480]
          frame #0 {
            n180 = VISA Write(VISA resource name=w476, write buffer=w478, error in (no error)=w477) -> (VISA resource name out=w474:refnum<visa-resource-name>, error out=w475:errorcluster)  [unwired: 1 out]
          }
          frame #1 {
            n181 = Wait (ms)(milliseconds to wait=u32 50) -> ()  [unwired: 1 out]
          }
        }
        n182 = VISA Clear(VISA resource name=w463, error in (no error)=w465) -> (VISA resource name out=w460:refnum<visa-resource-name>, error out=w464:errorcluster)
        n183 = local write "VISA resource name out"(w460) -> ()
      }
      event "BK1": Value Change {
        w495 = u16 0 items=["T0"=0, "A"=2, "B"=3, "C"=4, "D"=5, "E"=6, "F"=7, "G"=8, "H"=9] ("Reference Channel (0:T0)")
        w499 = u16 7 items=["A"=2, "B"=3, "C"=4, "D"=5, "E"=6, "F"=7, "G"=8, "H"=9] ("Channel to Modify (2:A)")
        n184 = event-data() -> ()  [unwired: 1 in, 6 out]
        n185 = Subtract(x="Delay F (0 s)", y=ext 100.0) -> (x-y=w483:ext)
        n186 = Divide(x=w483, y=ext 1000000000.0) -> (x/y=w482:ext)
        n187 = Format Into String(format string="%.;DLAY%d,%d,%.12g" ("Set Delay Command"), w499, w495, w482) -> (resulting string=w498:string)  [unwired: 2 in, 1 out]
        n188 = Concatenate Strings(w498, "\r\n") -> (w497:string)
        n189 = flat-sequence {
          tunnel: w497 -> [w505]
          tunnel: w494 -> [w504]
          tunnel: refnum<visa-resource-name> "DG645" ("VISA resource name") -> [w503]
          tunnel: [w502] -> w489
          tunnel: [w501] -> w488
          tunnel: [w507] -> w491
          tunnel: [w508] -> w492
          tunnel: w489 -> [w508]
          tunnel: w488 -> [w507]
          frame #0 {
            n190 = VISA Write(VISA resource name=w503, write buffer=w505, error in (no error)=w504) -> (VISA resource name out=w501:refnum<visa-resource-name>, error out=w502:errorcluster)  [unwired: 1 out]
          }
          frame #1 {
            n191 = Wait (ms)(milliseconds to wait=u32 50) -> ()  [unwired: 1 out]
          }
        }
        n192 = VISA Clear(VISA resource name=w491, error in (no error)=w492) -> (VISA resource name out=w487:refnum<visa-resource-name>, error out=w490:errorcluster)
        n193 = local write "VISA resource name out"(w487) -> ()
      }
      event "BK2": Value Change {
        w522 = u16 0 items=["T0"=0, "A"=2, "B"=3, "C"=4, "D"=5, "E"=6, "F"=7, "G"=8, "H"=9] ("Reference Channel (0:T0)")
        w526 = u16 8 items=["A"=2, "B"=3, "C"=4, "D"=5, "E"=6, "F"=7, "G"=8, "H"=9] ("Channel to Modify (2:A)")
        n194 = event-data() -> ()  [unwired: 1 in, 6 out]
        n195 = Subtract(x="Delay G (0 s)", y=ext 100.0) -> (x-y=w510:ext)
        n196 = Divide(x=w510, y=ext 1000000000.0) -> (x/y=w509:ext)
        n197 = Format Into String(format string="%.;DLAY%d,%d,%.12g" ("Set Delay Command"), w526, w522, w509) -> (resulting string=w525:string)  [unwired: 2 in, 1 out]
        n198 = Concatenate Strings(w525, "\r\n") -> (w524:string)
        n199 = flat-sequence {
          tunnel: w524 -> [w532]
          tunnel: w521 -> [w531]
          tunnel: refnum<visa-resource-name> "DG645" ("VISA resource name") -> [w530]
          tunnel: [w529] -> w516
          tunnel: [w528] -> w515
          tunnel: [w534] -> w517
          tunnel: [w535] -> w519
          tunnel: w516 -> [w535]
          tunnel: w515 -> [w534]
          frame #0 {
            n200 = VISA Write(VISA resource name=w530, write buffer=w532, error in (no error)=w531) -> (VISA resource name out=w528:refnum<visa-resource-name>, error out=w529:errorcluster)  [unwired: 1 out]
          }
          frame #1 {
            n201 = Wait (ms)(milliseconds to wait=u32 50) -> ()  [unwired: 1 out]
          }
        }
        n202 = VISA Clear(VISA resource name=w517, error in (no error)=w519) -> (VISA resource name out=w514:refnum<visa-resource-name>, error out=w518:errorcluster)
        n203 = local write "VISA resource name out"(w514) -> ()
      }
      event "BK3": Value Change {
        w549 = u16 0 items=["T0"=0, "A"=2, "B"=3, "C"=4, "D"=5, "E"=6, "F"=7, "G"=8, "H"=9] ("Reference Channel (0:T0)")
        w553 = u16 9 items=["A"=2, "B"=3, "C"=4, "D"=5, "E"=6, "F"=7, "G"=8, "H"=9] ("Channel to Modify (2:A)")
        n204 = event-data() -> ()  [unwired: 1 in, 6 out]
        n205 = Subtract(x="Delay H (0 s)", y=ext 100.0) -> (x-y=w537:ext)
        n206 = Divide(x=w537, y=ext 1000000000.0) -> (x/y=w536:ext)
        n207 = Format Into String(format string="%.;DLAY%d,%d,%.12g" ("Set Delay Command"), w553, w549, w536) -> (resulting string=w552:string)  [unwired: 2 in, 1 out]
        n208 = Concatenate Strings(w552, "\r\n") -> (w551:string)
        n209 = flat-sequence {
          tunnel: w551 -> [w559]
          tunnel: w548 -> [w558]
          tunnel: refnum<visa-resource-name> "DG645" ("VISA resource name") -> [w557]
          tunnel: [w556] -> w543
          tunnel: [w555] -> w542
          tunnel: [w561] -> w544
          tunnel: [w562] -> w546
          tunnel: w543 -> [w562]
          tunnel: w542 -> [w561]
          frame #0 {
            n210 = VISA Write(VISA resource name=w557, write buffer=w559, error in (no error)=w558) -> (VISA resource name out=w555:refnum<visa-resource-name>, error out=w556:errorcluster)  [unwired: 1 out]
          }
          frame #1 {
            n211 = Wait (ms)(milliseconds to wait=u32 50) -> ()  [unwired: 1 out]
          }
        }
        n212 = VISA Clear(VISA resource name=w544, error in (no error)=w546) -> (VISA resource name out=w541:refnum<visa-resource-name>, error out=w545:errorcluster)
        n213 = local write "VISA resource name out"(w541) -> ()
      }
      event "BZ2K1W": Value Change {
        n214 = event-data() -> ("NewVal"=w571:bool)  [unwired: 1 in]
        n215 = flat-sequence {
          tunnel: w571 -> [w576]
          tunnel: w570 -> [w575]
          tunnel: refnum<visa-resource-name> "COM1" ("VISA resource name") -> [w574]
          tunnel: [w573] -> w565
          tunnel: [w572] -> w564
          tunnel: [w592] -> w567
          tunnel: [w593] -> w568
          tunnel: w565 -> [w593]
          tunnel: w564 -> [w592]
          frame #0 {
            n216 = case shown="True" w576 {
              tunnel: [w580 w587] -> w572
              tunnel: [w579 w586] -> w573
              tunnel: w575 -> [w578 w585]
              tunnel: w574 -> [w577 w584]
              frame False {
                n217 = Concatenate Strings("#041000" ("string"), "\r\n") -> (w583:string)
                n218 = VISA Write(VISA resource name=w577, write buffer=w583, error in (no error)=w578) -> (VISA resource name out=w580:refnum<visa-resource-name>, error out=w579:errorcluster)  [unwired: 1 out]
              }
              frame True {
                n219 = Concatenate Strings("#041001" ("string"), "\r\n") -> (w590:string)
                n220 = VISA Write(VISA resource name=w584, write buffer=w590, error in (no error)=w585) -> (VISA resource name out=w587:refnum<visa-resource-name>, error out=w586:errorcluster)  [unwired: 1 out]
              }
            }
          }
          frame #1 {
            n221 = Wait (ms)(milliseconds to wait=u32 50) -> ()  [unwired: 1 out]
          }
        }
        n222 = VISA Clear(VISA resource name=w567, error in (no error)=w568) -> (VISA resource name out=w563:refnum<visa-resource-name>, error out=w566:errorcluster)
        n223 = local write "VISA resource name out"(w563) -> ()
      }
      event "DZ1K2W": Value Change {
        n224 = event-data() -> ("NewVal"=w600:bool)  [unwired: 1 in]
        n225 = flat-sequence {
          tunnel: w600 -> [w605]
          tunnel: refnum<visa-resource-name> "COM1" ("VISA resource name") -> [w604]
          tunnel: w598 -> [w603]
          tunnel: [w607] -> w596
          tunnel: [w606] -> w595
          tunnel: [w623] -> w601
          tunnel: [w624] -> w602
          tunnel: w596 -> [w624]
          tunnel: w595 -> [w623]
          frame #0 {
            n226 = case shown="True" w605 {
              tunnel: [w611 w618] -> w607
              tunnel: [w610 w617] -> w606
              tunnel: w603 -> [w609 w616]
              tunnel: w604 -> [w608 w615]
              frame False {
                n227 = Concatenate Strings("#041100" ("string"), "\r\n") -> (w614:string)
                n228 = VISA Write(VISA resource name=w608, write buffer=w614, error in (no error)=w609) -> (VISA resource name out=w610:refnum<visa-resource-name>, error out=w611:errorcluster)  [unwired: 1 out]
              }
              frame True {
                n229 = Concatenate Strings("#041101" ("string"), "\r\n") -> (w621:string)
                n230 = VISA Write(VISA resource name=w615, write buffer=w621, error in (no error)=w616) -> (VISA resource name out=w617:refnum<visa-resource-name>, error out=w618:errorcluster)  [unwired: 1 out]
              }
            }
          }
          frame #1 {
            n231 = Wait (ms)(milliseconds to wait=u32 50) -> ()  [unwired: 1 out]
          }
        }
        n232 = VISA Clear(VISA resource name=w601, error in (no error)=w602) -> (VISA resource name out=w594:refnum<visa-resource-name>, error out=w597:errorcluster)
        n233 = local write "VISA resource name out"(w594) -> ()
      }
      event "DZ2K2W": Value Change {
        n234 = event-data() -> ("NewVal"=w633:bool)  [unwired: 1 in]
        n235 = flat-sequence {
          tunnel: w633 -> [w638]
          tunnel: refnum<visa-resource-name> "COM1" ("VISA resource name") -> [w637]
          tunnel: w631 -> [w636]
          tunnel: [w635] -> w627
          tunnel: [w634] -> w626
          tunnel: [w654] -> w629
          tunnel: [w655] -> w630
          tunnel: w627 -> [w655]
          tunnel: w626 -> [w654]
          frame #0 {
            n236 = case shown="True" w638 {
              tunnel: [w640 w649] -> w635
              tunnel: [w639 w648] -> w634
              tunnel: w637 -> [w642 w647]
              tunnel: w636 -> [w641 w646]
              frame False {
                n237 = Concatenate Strings("#041200" ("string"), "\r\n") -> (w645:string)
                n238 = VISA Write(VISA resource name=w642, write buffer=w645, error in (no error)=w641) -> (VISA resource name out=w639:refnum<visa-resource-name>, error out=w640:errorcluster)  [unwired: 1 out]
              }
              frame True {
                n239 = Concatenate Strings("#041201" ("string"), "\r\n") -> (w652:string)
                n240 = VISA Write(VISA resource name=w647, write buffer=w652, error in (no error)=w646) -> (VISA resource name out=w648:refnum<visa-resource-name>, error out=w649:errorcluster)  [unwired: 1 out]
              }
            }
          }
          frame #1 {
            n241 = Wait (ms)(milliseconds to wait=u32 50) -> ()  [unwired: 1 out]
          }
        }
        n242 = VISA Clear(VISA resource name=w629, error in (no error)=w630) -> (VISA resource name out=w625:refnum<visa-resource-name>, error out=w628:errorcluster)
        n243 = local write "VISA resource name out"(w625) -> ()
      }
      event "BZ1K2W": Value Change {
        n244 = event-data() -> ("NewVal"=w664:bool)  [unwired: 1 in]
        n245 = flat-sequence {
          tunnel: w664 -> [w669]
          tunnel: refnum<visa-resource-name> "COM1" ("VISA resource name") -> [w668]
          tunnel: w662 -> [w667]
          tunnel: [w666] -> w658
          tunnel: [w665] -> w657
          tunnel: [w685] -> w660
          tunnel: [w686] -> w661
          tunnel: w658 -> [w686]
          tunnel: w657 -> [w685]
          frame #0 {
            n246 = case shown="True" w669 {
              tunnel: w668 -> [w673 w680]
              tunnel: w667 -> [w672 w679]
              tunnel: [w671 w677] -> w666
              tunnel: [w670 w678] -> w665
              frame False {
                n247 = Concatenate Strings("#041300" ("string"), "\r\n") -> (w676:string)
                n248 = VISA Write(VISA resource name=w673, write buffer=w676, error in (no error)=w672) -> (VISA resource name out=w670:refnum<visa-resource-name>, error out=w671:errorcluster)  [unwired: 1 out]
              }
              frame True {
                n249 = Concatenate Strings("#041301" ("string"), "\r\n") -> (w683:string)
                n250 = VISA Write(VISA resource name=w680, write buffer=w683, error in (no error)=w679) -> (VISA resource name out=w678:refnum<visa-resource-name>, error out=w677:errorcluster)  [unwired: 1 out]
              }
            }
          }
          frame #1 {
            n251 = Wait (ms)(milliseconds to wait=u32 50) -> ()  [unwired: 1 out]
          }
        }
        n252 = VISA Clear(VISA resource name=w660, error in (no error)=w661) -> (VISA resource name out=w656:refnum<visa-resource-name>, error out=w659:errorcluster)
        n253 = local write "VISA resource name out"(w656) -> ()
      }
      event "BZ2K2W": Value Change {
        n254 = event-data() -> ("NewVal"=w695:bool)  [unwired: 1 in]
        n255 = flat-sequence {
          tunnel: w695 -> [w700]
          tunnel: refnum<visa-resource-name> "COM1" ("VISA resource name") -> [w699]
          tunnel: w693 -> [w698]
          tunnel: [w697] -> w689
          tunnel: [w696] -> w688
          tunnel: [w716] -> w690
          tunnel: [w717] -> w692
          tunnel: w689 -> [w717]
          tunnel: w688 -> [w716]
          frame #0 {
            n256 = case shown="True" w700 {
              tunnel: [w702 w711] -> w697
              tunnel: [w701 w710] -> w696
              tunnel: w698 -> [w704 w709]
              tunnel: w699 -> [w703 w708]
              frame False {
                n257 = Concatenate Strings("#041400" ("string"), "\r\n") -> (w707:string)
                n258 = VISA Write(VISA resource name=w703, write buffer=w707, error in (no error)=w704) -> (VISA resource name out=w701:refnum<visa-resource-name>, error out=w702:errorcluster)  [unwired: 1 out]
              }
              frame True {
                n259 = Concatenate Strings("#041401" ("string"), "\r\n") -> (w714:string)
                n260 = VISA Write(VISA resource name=w708, write buffer=w714, error in (no error)=w709) -> (VISA resource name out=w710:refnum<visa-resource-name>, error out=w711:errorcluster)  [unwired: 1 out]
              }
            }
          }
          frame #1 {
            n261 = Wait (ms)(milliseconds to wait=u32 50) -> ()  [unwired: 1 out]
          }
        }
        n262 = VISA Clear(VISA resource name=w690, error in (no error)=w692) -> (VISA resource name out=w687:refnum<visa-resource-name>, error out=w691:errorcluster)
        n263 = local write "VISA resource name out"(w687) -> ()
      }
      event "DZ1K1W": Value Change {
        n264 = event-data() -> ("NewVal"=w726:bool)  [unwired: 1 in]
        n265 = flat-sequence {
          tunnel: w726 -> [w731]
          tunnel: refnum<visa-resource-name> "COM1" ("VISA resource name") -> [w730]
          tunnel: w724 -> [w729]
          tunnel: [w728] -> w720
          tunnel: [w727] -> w719
          tunnel: [w747] -> w722
          tunnel: [w748] -> w723
          tunnel: w720 -> [w748]
          tunnel: w719 -> [w747]
          frame #0 {
            n266 = case shown="True" w731 {
              tunnel: [w735 w742] -> w728
              tunnel: [w734 w741] -> w727
              tunnel: w730 -> [w733 w739]
              tunnel: w729 -> [w732 w740]
              frame False {
                n267 = Concatenate Strings("#041500" ("string"), "\r\n") -> (w738:string)
                n268 = VISA Write(VISA resource name=w733, write buffer=w738, error in (no error)=w732) -> (VISA resource name out=w734:refnum<visa-resource-name>, error out=w735:errorcluster)  [unwired: 1 out]
              }
              frame True {
                n269 = Concatenate Strings("#041501" ("string"), "\r\n") -> (w745:string)
                n270 = VISA Write(VISA resource name=w739, write buffer=w745, error in (no error)=w740) -> (VISA resource name out=w741:refnum<visa-resource-name>, error out=w742:errorcluster)  [unwired: 1 out]
              }
            }
          }
          frame #1 {
            n271 = Wait (ms)(milliseconds to wait=u32 50) -> ()  [unwired: 1 out]
          }
        }
        n272 = VISA Clear(VISA resource name=w722, error in (no error)=w723) -> (VISA resource name out=w718:refnum<visa-resource-name>, error out=w721:errorcluster)
        n273 = local write "VISA resource name out"(w718) -> ()
      }
      event "DZ2K1W": Value Change {
        n274 = event-data() -> ("NewVal"=w757:bool)  [unwired: 1 in]
        n275 = flat-sequence {
          tunnel: w757 -> [w762]
          tunnel: refnum<visa-resource-name> "COM1" ("VISA resource name") -> [w761]
          tunnel: w755 -> [w760]
          tunnel: [w759] -> w751
          tunnel: [w758] -> w750
          tunnel: [w778] -> w752
          tunnel: [w779] -> w754
          tunnel: w751 -> [w779]
          tunnel: w750 -> [w778]
          frame #0 {
            n276 = case shown="True" w762 {
              tunnel: [w766 w772] -> w759
              tunnel: [w765 w773] -> w758
              tunnel: w760 -> [w764 w771]
              tunnel: w761 -> [w763 w770]
              frame False {
                n277 = Concatenate Strings("#041600" ("string"), "\r\n") -> (w769:string)
                n278 = VISA Write(VISA resource name=w763, write buffer=w769, error in (no error)=w764) -> (VISA resource name out=w765:refnum<visa-resource-name>, error out=w766:errorcluster)  [unwired: 1 out]
              }
              frame True {
                n279 = Concatenate Strings("#041601" ("string"), "\r\n") -> (w776:string)
                n280 = VISA Write(VISA resource name=w770, write buffer=w776, error in (no error)=w771) -> (VISA resource name out=w773:refnum<visa-resource-name>, error out=w772:errorcluster)  [unwired: 1 out]
              }
            }
          }
          frame #1 {
            n281 = Wait (ms)(milliseconds to wait=u32 50) -> ()  [unwired: 1 out]
          }
        }
        n282 = VISA Clear(VISA resource name=w752, error in (no error)=w754) -> (VISA resource name out=w749:refnum<visa-resource-name>, error out=w753:errorcluster)
        n283 = local write "VISA resource name out"(w749) -> ()
      }
      event "BZ1K1W": Value Change {
        n284 = event-data() -> ("NewVal"=w788:bool)  [unwired: 1 in]
        n285 = flat-sequence {
          tunnel: w788 -> [w793]
          tunnel: refnum<visa-resource-name> "COM1" ("VISA resource name") -> [w792]
          tunnel: w786 -> [w791]
          tunnel: [w790] -> w782
          tunnel: [w789] -> w781
          tunnel: [w809] -> w784
          tunnel: [w810] -> w785
          tunnel: w782 -> [w810]
          tunnel: w781 -> [w809]
          frame #0 {
            n286 = case shown="True" w793 {
              tunnel: w791 -> [w797 w801]
              tunnel: w792 -> [w796 w802]
              tunnel: [w795 w804] -> w790
              tunnel: [w794 w803] -> w789
              frame False {
                n287 = Concatenate Strings("#041700" ("string"), "\r\n") -> (w800:string)
                n288 = VISA Write(VISA resource name=w796, write buffer=w800, error in (no error)=w797) -> (VISA resource name out=w794:refnum<visa-resource-name>, error out=w795:errorcluster)  [unwired: 1 out]
              }
              frame True {
                n289 = Concatenate Strings("#041701" ("string"), "\r\n") -> (w807:string)
                n290 = VISA Write(VISA resource name=w802, write buffer=w807, error in (no error)=w801) -> (VISA resource name out=w803:refnum<visa-resource-name>, error out=w804:errorcluster)  [unwired: 1 out]
              }
            }
          }
          frame #1 {
            n291 = Wait (ms)(milliseconds to wait=u32 50) -> ()  [unwired: 1 out]
          }
        }
        n292 = VISA Clear(VISA resource name=w784, error in (no error)=w785) -> (VISA resource name out=w780:refnum<visa-resource-name>, error out=w783:errorcluster)
        n293 = local write "VISA resource name out"(w780) -> ()
      }
      event "GF": Value Change {
        n294 = event-data() -> ("NewVal"=w819:bool)  [unwired: 1 in]
        n295 = flat-sequence {
          tunnel: w819 -> [w824]
          tunnel: refnum<visa-resource-name> "COM1" ("VISA resource name") -> [w823]
          tunnel: w817 -> [w822]
          tunnel: [w821] -> w813
          tunnel: [w820] -> w812
          tunnel: [w840] -> w815
          tunnel: [w841] -> w816
          tunnel: w813 -> [w841]
          tunnel: w812 -> [w840]
          frame #0 {
            n296 = case shown="True" w824 {
              tunnel: [w828 w835] -> w820
              tunnel: [w827 w834] -> w821
              tunnel: w822 -> [w826 w833]
              tunnel: w823 -> [w825 w832]
              frame False {
                n297 = Concatenate Strings("#051000" ("string"), "\r\n") -> (w831:string)
                n298 = VISA Write(VISA resource name=w825, write buffer=w831, error in (no error)=w826) -> (VISA resource name out=w828:refnum<visa-resource-name>, error out=w827:errorcluster)  [unwired: 1 out]
              }
              frame True {
                n299 = Concatenate Strings("#051001" ("string"), "\r\n") -> (w838:string)
                n300 = VISA Write(VISA resource name=w832, write buffer=w838, error in (no error)=w833) -> (VISA resource name out=w835:refnum<visa-resource-name>, error out=w834:errorcluster)  [unwired: 1 out]
              }
            }
          }
          frame #1 {
            n301 = Wait (ms)(milliseconds to wait=u32 50) -> ()  [unwired: 1 out]
          }
        }
        n302 = VISA Clear(VISA resource name=w815, error in (no error)=w816) -> (VISA resource name out=w811:refnum<visa-resource-name>, error out=w814:errorcluster)
        n303 = local write "VISA resource name out"(w811) -> ()
      }
      event "Kamera Y": Value Change {
        n304 = event-data() -> ("NewVal"=w850:bool)  [unwired: 1 in]
        n305 = flat-sequence {
          tunnel: w850 -> [w855]
          tunnel: w849 -> [w854]
          tunnel: refnum<visa-resource-name> "COM1" ("VISA resource name") -> [w853]
          tunnel: [w852] -> w844
          tunnel: [w851] -> w843
          tunnel: [w871] -> w846
          tunnel: [w872] -> w847
          tunnel: w844 -> [w872]
          tunnel: w843 -> [w871]
          frame #0 {
            n306 = case shown="True" w855 {
              tunnel: [w859 w866] -> w852
              tunnel: [w858 w865] -> w851
              tunnel: w854 -> [w857 w864]
              tunnel: w853 -> [w856 w863]
              frame False {
                n307 = Concatenate Strings("#051100" ("string"), "\r\n") -> (w862:string)
                n308 = VISA Write(VISA resource name=w856, write buffer=w862, error in (no error)=w857) -> (VISA resource name out=w858:refnum<visa-resource-name>, error out=w859:errorcluster)  [unwired: 1 out]
              }
              frame True {
                n309 = Concatenate Strings("#051101" ("string"), "\r\n") -> (w869:string)
                n310 = VISA Write(VISA resource name=w863, write buffer=w869, error in (no error)=w864) -> (VISA resource name out=w865:refnum<visa-resource-name>, error out=w866:errorcluster)  [unwired: 1 out]
              }
            }
          }
          frame #1 {
            n311 = Wait (ms)(milliseconds to wait=u32 50) -> ()  [unwired: 1 out]
          }
        }
        n312 = VISA Clear(VISA resource name=w846, error in (no error)=w847) -> (VISA resource name out=w842:refnum<visa-resource-name>, error out=w845:errorcluster)
        n313 = local write "VISA resource name out"(w842) -> ()
      }
      event "BK1": Value Change {
        n314 = event-data() -> ("NewVal"=w881:bool)  [unwired: 1 in]
        n315 = flat-sequence {
          tunnel: w881 -> [w886]
          tunnel: refnum<visa-resource-name> "COM1" ("VISA resource name") -> [w885]
          tunnel: w879 -> [w884]
          tunnel: [w883] -> w875
          tunnel: [w882] -> w874
          tunnel: [w902] -> w877
          tunnel: [w903] -> w878
          tunnel: w875 -> [w903]
          tunnel: w874 -> [w902]
          frame #0 {
            n316 = case shown="True" w886 {
              tunnel: [w888 w897] -> w883
              tunnel: [w887 w896] -> w882
              tunnel: w885 -> [w890 w895]
              tunnel: w884 -> [w889 w894]
              frame False {
                n317 = Concatenate Strings("#051200" ("string"), "\r\n") -> (w893:string)
                n318 = VISA Write(VISA resource name=w890, write buffer=w893, error in (no error)=w889) -> (VISA resource name out=w887:refnum<visa-resource-name>, error out=w888:errorcluster)  [unwired: 1 out]
              }
              frame True {
                n319 = Concatenate Strings("#051201" ("string"), "\r\n") -> (w900:string)
                n320 = VISA Write(VISA resource name=w895, write buffer=w900, error in (no error)=w894) -> (VISA resource name out=w896:refnum<visa-resource-name>, error out=w897:errorcluster)  [unwired: 1 out]
              }
            }
          }
          frame #1 {
            n321 = Wait (ms)(milliseconds to wait=u32 50) -> ()  [unwired: 1 out]
          }
        }
        n322 = VISA Clear(VISA resource name=w877, error in (no error)=w878) -> (VISA resource name out=w873:refnum<visa-resource-name>, error out=w876:errorcluster)
        n323 = local write "VISA resource name out"(w873) -> ()
      }
      event "BK 2": Value Change {
        n324 = event-data() -> ("NewVal"=w912:bool)  [unwired: 1 in]
        n325 = flat-sequence {
          tunnel: w912 -> [w917]
          tunnel: refnum<visa-resource-name> "COM1" ("VISA resource name") -> [w916]
          tunnel: w910 -> [w915]
          tunnel: [w914] -> w906
          tunnel: [w913] -> w905
          tunnel: [w933] -> w908
          tunnel: [w934] -> w909
          tunnel: w906 -> [w934]
          tunnel: w905 -> [w933]
          frame #0 {
            n326 = case shown="True" w917 {
              tunnel: w916 -> [w921 w928]
              tunnel: w915 -> [w920 w927]
              tunnel: [w919 w925] -> w914
              tunnel: [w918 w926] -> w913
              frame False {
                n327 = Concatenate Strings("#051300" ("string"), "\r\n") -> (w924:string)
                n328 = VISA Write(VISA resource name=w921, write buffer=w924, error in (no error)=w920) -> (VISA resource name out=w918:refnum<visa-resource-name>, error out=w919:errorcluster)  [unwired: 1 out]
              }
              frame True {
                n329 = Concatenate Strings("#051301" ("string"), "\r\n") -> (w931:string)
                n330 = VISA Write(VISA resource name=w928, write buffer=w931, error in (no error)=w927) -> (VISA resource name out=w926:refnum<visa-resource-name>, error out=w925:errorcluster)  [unwired: 1 out]
              }
            }
          }
          frame #1 {
            n331 = Wait (ms)(milliseconds to wait=u32 50) -> ()  [unwired: 1 out]
          }
        }
        n332 = VISA Clear(VISA resource name=w908, error in (no error)=w909) -> (VISA resource name out=w904:refnum<visa-resource-name>, error out=w907:errorcluster)
        n333 = local write "VISA resource name out"(w904) -> ()
      }
      event "BK3": Value Change {
        n334 = event-data() -> ("NewVal"=w943:bool)  [unwired: 1 in]
        n335 = flat-sequence {
          tunnel: w943 -> [w948]
          tunnel: refnum<visa-resource-name> "COM1" ("VISA resource name") -> [w947]
          tunnel: w941 -> [w946]
          tunnel: [w945] -> w937
          tunnel: [w944] -> w936
          tunnel: [w964] -> w939
          tunnel: [w965] -> w940
          tunnel: w937 -> [w965]
          tunnel: w936 -> [w964]
          frame #0 {
            n336 = case shown="True" w948 {
              tunnel: [w950 w959] -> w945
              tunnel: [w949 w958] -> w944
              tunnel: w946 -> [w952 w957]
              tunnel: w947 -> [w951 w956]
              frame False {
                n337 = Concatenate Strings("#051400" ("string"), "\r\n") -> (w955:string)
                n338 = VISA Write(VISA resource name=w951, write buffer=w955, error in (no error)=w952) -> (VISA resource name out=w949:refnum<visa-resource-name>, error out=w950:errorcluster)  [unwired: 1 out]
              }
              frame True {
                n339 = Concatenate Strings("#051401" ("string"), "\r\n") -> (w962:string)
                n340 = VISA Write(VISA resource name=w956, write buffer=w962, error in (no error)=w957) -> (VISA resource name out=w958:refnum<visa-resource-name>, error out=w959:errorcluster)  [unwired: 1 out]
              }
            }
          }
          frame #1 {
            n341 = Wait (ms)(milliseconds to wait=u32 50) -> ()  [unwired: 1 out]
          }
        }
        n342 = VISA Clear(VISA resource name=w939, error in (no error)=w940) -> (VISA resource name out=w935:refnum<visa-resource-name>, error out=w938:errorcluster)
        n343 = local write "VISA resource name out"(w935) -> ()
      }
      event "F-R VISAR 4": Value Change {
        n344 = event-data() -> ("NewVal"=w974:bool)  [unwired: 1 in]
        n345 = flat-sequence {
          tunnel: w974 -> [w979]
          tunnel: refnum<visa-resource-name> "COM1" ("VISA resource name") -> [w978]
          tunnel: w972 -> [w977]
          tunnel: [w976] -> w968
          tunnel: [w975] -> w967
          tunnel: [w995] -> w970
          tunnel: [w996] -> w971
          tunnel: w968 -> [w996]
          tunnel: w967 -> [w995]
          frame #0 {
            n346 = case shown="True" w979 {
              tunnel: [w983 w990] -> w976
              tunnel: [w982 w989] -> w975
              tunnel: w978 -> [w981 w987]
              tunnel: w977 -> [w980 w988]
              frame False {
                n347 = Concatenate Strings("#051500" ("string"), "\r\n") -> (w986:string)
                n348 = VISA Write(VISA resource name=w981, write buffer=w986, error in (no error)=w980) -> (VISA resource name out=w982:refnum<visa-resource-name>, error out=w983:errorcluster)  [unwired: 1 out]
              }
              frame True {
                n349 = Concatenate Strings("#051501" ("string"), "\r\n") -> (w993:string)
                n350 = VISA Write(VISA resource name=w987, write buffer=w993, error in (no error)=w988) -> (VISA resource name out=w989:refnum<visa-resource-name>, error out=w990:errorcluster)  [unwired: 1 out]
              }
            }
          }
          frame #1 {
            n351 = Wait (ms)(milliseconds to wait=u32 50) -> ()  [unwired: 1 out]
          }
        }
        n352 = VISA Clear(VISA resource name=w970, error in (no error)=w971) -> (VISA resource name out=w966:refnum<visa-resource-name>, error out=w969:errorcluster)
        n353 = local write "VISA resource name out"(w966) -> ()
      }
      event "F-R VISAR 3": Value Change {
        n354 = event-data() -> ("NewVal"=w1005:bool)  [unwired: 1 in]
        n355 = flat-sequence {
          tunnel: w1005 -> [w1010]
          tunnel: refnum<visa-resource-name> "COM1" ("VISA resource name") -> [w1009]
          tunnel: w1003 -> [w1008]
          tunnel: [w1007] -> w999
          tunnel: [w1006] -> w998
          tunnel: [w1026] -> w1001
          tunnel: [w1027] -> w1002
          tunnel: w999 -> [w1027]
          tunnel: w998 -> [w1026]
          frame #0 {
            n356 = case shown="True" w1010 {
              tunnel: [w1014 w1020] -> w1007
              tunnel: [w1013 w1021] -> w1006
              tunnel: w1008 -> [w1012 w1019]
              tunnel: w1009 -> [w1011 w1018]
              frame False {
                n357 = Concatenate Strings("#051600" ("string"), "\r\n") -> (w1017:string)
                n358 = VISA Write(VISA resource name=w1011, write buffer=w1017, error in (no error)=w1012) -> (VISA resource name out=w1013:refnum<visa-resource-name>, error out=w1014:errorcluster)  [unwired: 1 out]
              }
              frame True {
                n359 = Concatenate Strings("#051601" ("string"), "\r\n") -> (w1024:string)
                n360 = VISA Write(VISA resource name=w1018, write buffer=w1024, error in (no error)=w1019) -> (VISA resource name out=w1021:refnum<visa-resource-name>, error out=w1020:errorcluster)  [unwired: 1 out]
              }
            }
          }
          frame #1 {
            n361 = Wait (ms)(milliseconds to wait=u32 50) -> ()  [unwired: 1 out]
          }
        }
        n362 = VISA Clear(VISA resource name=w1001, error in (no error)=w1002) -> (VISA resource name out=w997:refnum<visa-resource-name>, error out=w1000:errorcluster)
        n363 = local write "VISA resource name out"(w997) -> ()
      }
      event "FI": Value Change {
        n364 = event-data() -> ("NewVal"=w1036:bool)  [unwired: 1 in]
        n365 = flat-sequence {
          tunnel: w1036 -> [w1041]
          tunnel: w1035 -> [w1040]
          tunnel: refnum<visa-resource-name> "COM1" ("VISA resource name") -> [w1039]
          tunnel: [w1038] -> w1030
          tunnel: [w1037] -> w1029
          tunnel: [w1057] -> w1032
          tunnel: [w1058] -> w1033
          tunnel: w1030 -> [w1058]
          tunnel: w1029 -> [w1057]
          frame #0 {
            n366 = case shown="True" w1041 {
              tunnel: w1040 -> [w1045 w1049]
              tunnel: w1039 -> [w1044 w1050]
              tunnel: [w1043 w1052] -> w1038
              tunnel: [w1042 w1051] -> w1037
              frame False {
                n367 = Concatenate Strings("#051700" ("string"), "\r\n") -> (w1048:string)
                n368 = VISA Write(VISA resource name=w1044, write buffer=w1048, error in (no error)=w1045) -> (VISA resource name out=w1042:refnum<visa-resource-name>, error out=w1043:errorcluster)  [unwired: 1 out]
              }
              frame True {
                n369 = Concatenate Strings("#051701" ("string"), "\r\n") -> (w1055:string)
                n370 = VISA Write(VISA resource name=w1050, write buffer=w1055, error in (no error)=w1049) -> (VISA resource name out=w1051:refnum<visa-resource-name>, error out=w1052:errorcluster)  [unwired: 1 out]
              }
            }
          }
          frame #1 {
            n371 = Wait (ms)(milliseconds to wait=u32 50) -> ()  [unwired: 1 out]
          }
        }
        n372 = VISA Clear(VISA resource name=w1032, error in (no error)=w1033) -> (VISA resource name out=w1028:refnum<visa-resource-name>, error out=w1031:errorcluster)
        n373 = local write "VISA resource name out"(w1028) -> ()
      }
      event "rele 0_6": Value Change {
        n374 = event-data() -> ("NewVal"=w1067:bool)  [unwired: 1 in]
        n375 = flat-sequence {
          tunnel: w1067 -> [w1072]
          tunnel: refnum<visa-resource-name> "COM1" ("VISA resource name") -> [w1071]
          tunnel: w1065 -> [w1070]
          tunnel: [w1069] -> w1061
          tunnel: [w1068] -> w1060
          tunnel: [w1088] -> w1063
          tunnel: [w1089] -> w1064
          tunnel: w1061 -> [w1089]
          tunnel: w1060 -> [w1088]
          frame #0 {
            n376 = case shown="True" w1072 {
              tunnel: [w1076 w1083] -> w1068
              tunnel: [w1075 w1082] -> w1069
              tunnel: w1070 -> [w1074 w1081]
              tunnel: w1071 -> [w1073 w1080]
              frame False {
                n377 = Concatenate Strings("#061000" ("string"), "\r\n") -> (w1079:string)
                n378 = VISA Write(VISA resource name=w1073, write buffer=w1079, error in (no error)=w1074) -> (VISA resource name out=w1076:refnum<visa-resource-name>, error out=w1075:errorcluster)  [unwired: 1 out]
              }
              frame True {
                n379 = Concatenate Strings("#061001" ("string"), "\r\n") -> (w1086:string)
                n380 = VISA Write(VISA resource name=w1080, write buffer=w1086, error in (no error)=w1081) -> (VISA resource name out=w1083:refnum<visa-resource-name>, error out=w1082:errorcluster)  [unwired: 1 out]
              }
            }
          }
          frame #1 {
            n381 = Wait (ms)(milliseconds to wait=u32 50) -> ()  [unwired: 1 out]
          }
        }
        n382 = VISA Clear(VISA resource name=w1063, error in (no error)=w1064) -> (VISA resource name out=w1059:refnum<visa-resource-name>, error out=w1062:errorcluster)
        n383 = local write "VISA resource name out"(w1059) -> ()
      }
      event "F0-ethernet 4": Value Change {
        n384 = event-data() -> ("NewVal"=w1098:bool)  [unwired: 1 in]
        n385 = flat-sequence {
          tunnel: w1098 -> [w1103]
          tunnel: refnum<visa-resource-name> "COM1" ("VISA resource name") -> [w1102]
          tunnel: w1096 -> [w1101]
          tunnel: [w1100] -> w1092
          tunnel: [w1099] -> w1091
          tunnel: [w1119] -> w1094
          tunnel: [w1120] -> w1095
          tunnel: w1092 -> [w1120]
          tunnel: w1091 -> [w1119]
          frame #0 {
            n386 = case shown="True" w1103 {
              tunnel: [w1107 w1114] -> w1100
              tunnel: [w1106 w1113] -> w1099
              tunnel: w1101 -> [w1105 w1112]
              tunnel: w1102 -> [w1104 w1111]
              frame False {
                n387 = Concatenate Strings("#061100" ("string"), "\r\n") -> (w1110:string)
                n388 = VISA Write(VISA resource name=w1104, write buffer=w1110, error in (no error)=w1105) -> (VISA resource name out=w1106:refnum<visa-resource-name>, error out=w1107:errorcluster)  [unwired: 1 out]
              }
              frame True {
                n389 = Concatenate Strings("#061101" ("string"), "\r\n") -> (w1117:string)
                n390 = VISA Write(VISA resource name=w1111, write buffer=w1117, error in (no error)=w1112) -> (VISA resource name out=w1113:refnum<visa-resource-name>, error out=w1114:errorcluster)  [unwired: 1 out]
              }
            }
          }
          frame #1 {
            n391 = Wait (ms)(milliseconds to wait=u32 50) -> ()  [unwired: 1 out]
          }
        }
        n392 = VISA Clear(VISA resource name=w1094, error in (no error)=w1095) -> (VISA resource name out=w1090:refnum<visa-resource-name>, error out=w1093:errorcluster)
        n393 = local write "VISA resource name out"(w1090) -> ()
      }
      event "F0-ethernet 5": Value Change {
        n394 = event-data() -> ("NewVal"=w1129:bool)  [unwired: 1 in]
        n395 = flat-sequence {
          tunnel: w1129 -> [w1134]
          tunnel: refnum<visa-resource-name> "COM1" ("VISA resource name") -> [w1133]
          tunnel: w1127 -> [w1132]
          tunnel: [w1131] -> w1123
          tunnel: [w1130] -> w1122
          tunnel: [w1150] -> w1125
          tunnel: [w1151] -> w1126
          tunnel: w1123 -> [w1151]
          tunnel: w1122 -> [w1150]
          frame #0 {
            n396 = case shown="True" w1134 {
              tunnel: [w1136 w1145] -> w1131
              tunnel: [w1135 w1144] -> w1130
              tunnel: w1133 -> [w1138 w1143]
              tunnel: w1132 -> [w1137 w1142]
              frame False {
                n397 = Concatenate Strings("#061200" ("string"), "\r\n") -> (w1141:string)
                n398 = VISA Write(VISA resource name=w1138, write buffer=w1141, error in (no error)=w1137) -> (VISA resource name out=w1135:refnum<visa-resource-name>, error out=w1136:errorcluster)  [unwired: 1 out]
              }
              frame True {
                n399 = Concatenate Strings("#061201" ("string"), "\r\n") -> (w1148:string)
                n400 = VISA Write(VISA resource name=w1143, write buffer=w1148, error in (no error)=w1142) -> (VISA resource name out=w1144:refnum<visa-resource-name>, error out=w1145:errorcluster)  [unwired: 1 out]
              }
            }
          }
          frame #1 {
            n401 = Wait (ms)(milliseconds to wait=u32 50) -> ()  [unwired: 1 out]
          }
        }
        n402 = VISA Clear(VISA resource name=w1125, error in (no error)=w1126) -> (VISA resource name out=w1121:refnum<visa-resource-name>, error out=w1124:errorcluster)
        n403 = local write "VISA resource name out"(w1121) -> ()
      }
      event "F0-ethernet 1": Value Change {
        n404 = event-data() -> ("NewVal"=w1160:bool)  [unwired: 1 in]
        n405 = flat-sequence {
          tunnel: w1160 -> [w1165]
          tunnel: refnum<visa-resource-name> "COM1" ("VISA resource name") -> [w1164]
          tunnel: w1158 -> [w1163]
          tunnel: [w1162] -> w1154
          tunnel: [w1161] -> w1153
          tunnel: [w1181] -> w1156
          tunnel: [w1182] -> w1157
          tunnel: w1154 -> [w1182]
          tunnel: w1153 -> [w1181]
          frame #0 {
            n406 = case shown="True" w1165 {
              tunnel: w1164 -> [w1169 w1176]
              tunnel: w1163 -> [w1168 w1175]
              tunnel: [w1167 w1173] -> w1162
              tunnel: [w1166 w1174] -> w1161
              frame False {
                n407 = Concatenate Strings("#061300" ("string"), "\r\n") -> (w1172:string)
                n408 = VISA Write(VISA resource name=w1169, write buffer=w1172, error in (no error)=w1168) -> (VISA resource name out=w1166:refnum<visa-resource-name>, error out=w1167:errorcluster)  [unwired: 1 out]
              }
              frame True {
                n409 = Concatenate Strings("#061301" ("string"), "\r\n") -> (w1179:string)
                n410 = VISA Write(VISA resource name=w1176, write buffer=w1179, error in (no error)=w1175) -> (VISA resource name out=w1174:refnum<visa-resource-name>, error out=w1173:errorcluster)  [unwired: 1 out]
              }
            }
          }
          frame #1 {
            n411 = Wait (ms)(milliseconds to wait=u32 50) -> ()  [unwired: 1 out]
          }
        }
        n412 = VISA Clear(VISA resource name=w1156, error in (no error)=w1157) -> (VISA resource name out=w1152:refnum<visa-resource-name>, error out=w1155:errorcluster)
        n413 = local write "VISA resource name out"(w1152) -> ()
      }
      event "F0-ethernet 2": Value Change {
        n414 = event-data() -> ("NewVal"=w1191:bool)  [unwired: 1 in]
        n415 = flat-sequence {
          tunnel: w1191 -> [w1196]
          tunnel: refnum<visa-resource-name> "COM1" ("VISA resource name") -> [w1195]
          tunnel: w1189 -> [w1194]
          tunnel: [w1193] -> w1185
          tunnel: [w1192] -> w1184
          tunnel: [w1212] -> w1187
          tunnel: [w1213] -> w1188
          tunnel: w1185 -> [w1213]
          tunnel: w1184 -> [w1212]
          frame #0 {
            n416 = case shown="True" w1196 {
              tunnel: [w1198 w1207] -> w1193
              tunnel: [w1197 w1206] -> w1192
              tunnel: w1194 -> [w1200 w1205]
              tunnel: w1195 -> [w1199 w1204]
              frame False {
                n417 = Concatenate Strings("#061400" ("string"), "\r\n") -> (w1203:string)
                n418 = VISA Write(VISA resource name=w1199, write buffer=w1203, error in (no error)=w1200) -> (VISA resource name out=w1197:refnum<visa-resource-name>, error out=w1198:errorcluster)  [unwired: 1 out]
              }
              frame True {
                n419 = Concatenate Strings("#061401" ("string"), "\r\n") -> (w1210:string)
                n420 = VISA Write(VISA resource name=w1204, write buffer=w1210, error in (no error)=w1205) -> (VISA resource name out=w1206:refnum<visa-resource-name>, error out=w1207:errorcluster)  [unwired: 1 out]
              }
            }
          }
          frame #1 {
            n421 = Wait (ms)(milliseconds to wait=u32 50) -> ()  [unwired: 1 out]
          }
        }
        n422 = VISA Clear(VISA resource name=w1187, error in (no error)=w1188) -> (VISA resource name out=w1183:refnum<visa-resource-name>, error out=w1186:errorcluster)
        n423 = local write "VISA resource name out"(w1183) -> ()
      }
      event "PZS 1 DOP": Value Change {
        n424 = event-data() -> ("NewVal"=w1222:bool)  [unwired: 1 in]
        n425 = flat-sequence {
          tunnel: w1222 -> [w1227]
          tunnel: refnum<visa-resource-name> "COM1" ("VISA resource name") -> [w1226]
          tunnel: w1220 -> [w1225]
          tunnel: [w1224] -> w1216
          tunnel: [w1223] -> w1215
          tunnel: [w1243] -> w1218
          tunnel: [w1244] -> w1219
          tunnel: w1216 -> [w1244]
          tunnel: w1215 -> [w1243]
          frame #0 {
            n426 = case shown="True" w1227 {
              tunnel: [w1231 w1238] -> w1224
              tunnel: [w1230 w1237] -> w1223
              tunnel: w1226 -> [w1229 w1235]
              tunnel: w1225 -> [w1228 w1236]
              frame False {
                n427 = Concatenate Strings("#061500" ("string"), "\r\n") -> (w1234:string)
                n428 = VISA Write(VISA resource name=w1229, write buffer=w1234, error in (no error)=w1228) -> (VISA resource name out=w1230:refnum<visa-resource-name>, error out=w1231:errorcluster)  [unwired: 1 out]
              }
              frame True {
                n429 = Concatenate Strings("#061501" ("string"), "\r\n") -> (w1241:string)
                n430 = VISA Write(VISA resource name=w1235, write buffer=w1241, error in (no error)=w1236) -> (VISA resource name out=w1237:refnum<visa-resource-name>, error out=w1238:errorcluster)  [unwired: 1 out]
              }
            }
          }
          frame #1 {
            n431 = Wait (ms)(milliseconds to wait=u32 50) -> ()  [unwired: 1 out]
          }
        }
        n432 = VISA Clear(VISA resource name=w1218, error in (no error)=w1219) -> (VISA resource name out=w1214:refnum<visa-resource-name>, error out=w1217:errorcluster)
        n433 = local write "VISA resource name out"(w1214) -> ()
      }
      event "PZS 2 DOP": Value Change {
        n434 = event-data() -> ("NewVal"=w1253:bool)  [unwired: 1 in]
        n435 = flat-sequence {
          tunnel: w1253 -> [w1258]
          tunnel: refnum<visa-resource-name> "COM1" ("VISA resource name") -> [w1257]
          tunnel: w1251 -> [w1256]
          tunnel: [w1255] -> w1247
          tunnel: [w1254] -> w1246
          tunnel: [w1274] -> w1249
          tunnel: [w1275] -> w1250
          tunnel: w1247 -> [w1275]
          tunnel: w1246 -> [w1274]
          frame #0 {
            n436 = case shown="True" w1258 {
              tunnel: [w1262 w1268] -> w1255
              tunnel: [w1261 w1269] -> w1254
              tunnel: w1256 -> [w1260 w1267]
              tunnel: w1257 -> [w1259 w1266]
              frame False {
                n437 = Concatenate Strings("#061600" ("string"), "\r\n") -> (w1265:string)
                n438 = VISA Write(VISA resource name=w1259, write buffer=w1265, error in (no error)=w1260) -> (VISA resource name out=w1261:refnum<visa-resource-name>, error out=w1262:errorcluster)  [unwired: 1 out]
              }
              frame True {
                n439 = Concatenate Strings("#061601" ("string"), "\r\n") -> (w1272:string)
                n440 = VISA Write(VISA resource name=w1266, write buffer=w1272, error in (no error)=w1267) -> (VISA resource name out=w1269:refnum<visa-resource-name>, error out=w1268:errorcluster)  [unwired: 1 out]
              }
            }
          }
          frame #1 {
            n441 = Wait (ms)(milliseconds to wait=u32 50) -> ()  [unwired: 1 out]
          }
        }
        n442 = VISA Clear(VISA resource name=w1249, error in (no error)=w1250) -> (VISA resource name out=w1245:refnum<visa-resource-name>, error out=w1248:errorcluster)
        n443 = local write "VISA resource name out"(w1245) -> ()
      }
      event "F0-ethernet 3": Value Change {
        n444 = event-data() -> ("NewVal"=w1284:bool)  [unwired: 1 in]
        n445 = flat-sequence {
          tunnel: w1284 -> [w1289]
          tunnel: refnum<visa-resource-name> "COM1" ("VISA resource name") -> [w1288]
          tunnel: w1282 -> [w1287]
          tunnel: [w1286] -> w1278
          tunnel: [w1285] -> w1277
          tunnel: [w1305] -> w1280
          tunnel: [w1306] -> w1281
          tunnel: w1278 -> [w1306]
          tunnel: w1277 -> [w1305]
          frame #0 {
            n446 = case shown="True" w1289 {
              tunnel: w1287 -> [w1293 w1297]
              tunnel: w1288 -> [w1292 w1298]
              tunnel: [w1291 w1300] -> w1286
              tunnel: [w1290 w1299] -> w1285
              frame False {
                n447 = Concatenate Strings("#061700" ("string"), "\r\n") -> (w1296:string)
                n448 = VISA Write(VISA resource name=w1292, write buffer=w1296, error in (no error)=w1293) -> (VISA resource name out=w1290:refnum<visa-resource-name>, error out=w1291:errorcluster)  [unwired: 1 out]
              }
              frame True {
                n449 = Concatenate Strings("#061701" ("string"), "\r\n") -> (w1303:string)
                n450 = VISA Write(VISA resource name=w1298, write buffer=w1303, error in (no error)=w1297) -> (VISA resource name out=w1299:refnum<visa-resource-name>, error out=w1300:errorcluster)  [unwired: 1 out]
              }
            }
          }
          frame #1 {
            n451 = Wait (ms)(milliseconds to wait=u32 50) -> ()  [unwired: 1 out]
          }
        }
        n452 = VISA Clear(VISA resource name=w1280, error in (no error)=w1281) -> (VISA resource name out=w1276:refnum<visa-resource-name>, error out=w1279:errorcluster)
        n453 = local write "VISA resource name out"(w1276) -> ()
      }
    }
    "error out" <- w5
    "error out 2" <- w4
    n454 = VISA Close(VISA resource name=w10, error in (no error)=w5) -> (error out=w11:errorcluster)
    n455 = VISA Close(VISA resource name=w6, error in (no error)=w7) -> ()  [unwired: 1 out]
    n456 = VISA Close(VISA resource name=w9, error in (no error)=w8) -> ()  [unwired: 1 out]
  }
